vi "WildBugChilGru.vi"() -> ()   [LabVIEW 2014]
uses:
  <vilib>/Utility/miscctls.llb/LVPointTypeDef.ctl
  <vilib>/Utility/xml.llb/Write to XML File(string).vi
  <vilib>/Platform/browser.llb/Open URL in Default Browser (string).vi
  <vilib>/Instr/_visa.llb/VISA Configure Serial Port (Instr).vi
  <vilib>/Analysis/3filter.llb/IIR Filter (DBL).vi
  <vilib>/gmath/NI_Gmath.lvlib
  <vilib>/Analysis/NI_AALBase.lvlib
  <vilib>/ptbypt/NI_PtbyPt.lvlib
panel:
  out "Strecke [m]":dbl
  out "dT":dbl=3003.0
  out "Cyclecounter":dbl=3003.0
  out "Datum+Zeit":string="14.08.2020 22:16"
  out "n(Pmax)":dbl=5307.692307692308
  out "Pmax":dbl=17.77254327549455
  out "Lauf abgebrochen":bool
  out "Auto-Datei":string
  out "Auto-Gespeichert":bool
  in  "Auto-Pfad":path
  in  "Auto-Speichern":bool
  out "n(Rolle) [1/min]":dbl=3003.0
  in  "Fahrzeugdaten":string
  out "Ergebnis":string
  out "Pmax":string
  in  "Drucken":bool
  in  "Speichern":bool
  in  "Start":bool
  in  "Ende":bool
  in  "Spenden":bool
  in  "Registerkarte":T1(tab)
  in  "Zündung [Imp/U]":dbl=1.0 format="%#.2f"
  in  "Übersetzung ermitteln aus":T2(ring)
  in  "Getriebe [1:]":dbl=4.0 min=0.0001
  in  "Reifenumfang [m]":dbl=1.222 min=0.0001
  in  "Dauer [s]":u8=5
  in  "nKuWe/nRolle":dbl=20.0 format="%#.3f"
  in  "Lufttemperatur [°C]":dbl=23.3 format="%#.1g"
  in  "Luftdruck [mbar]":dbl=1013.45 min=0.0001
  in  "Messung Klimadaten":bool=TRUE
  in  "Filter Zündsignal":bool
  in  "v vom Gas [km/h]":u16=40
  in  "Gleitender Mittelwert":u8=35
  in  "Differenzenquotient":u8=12
  in  "n vom Gas [1/min]":u16=5000
  in  "Verlustmoment M1 [Nm] bei n1":dbl min=0.0
  in  "Rollendrehzahl n1 [1/min]":u16=1 min=1
  in  "Verlustmoment M0 [Nm] bei n = 0":dbl min=0.0
  in  "Rollengeber [Inkr/U]":u16=20 min=1
  in  "Rollenumfang [m]":dbl=0.5 min=0.0001
  in  "Rollenträgheit [kgm²]":dbl=2.0 min=0.0001
  in  "Rollendrehzahl aufzeichnen":bool
  in  "Überschrift Leistungsdiagramm":string
  in  "Recalc":bool
  in  "Leistung":bool=TRUE caption="Messung Klimadaten"
  out "Datenspeicher":T3={"Fahrzeugdaten"="§$", "Auto-Pfad"="14.08.2020 22:16|", "Rolle [Inkr/U]"=20, "Rollenumfang [m]"=0.5, "Rollenträgheit [kgm²]"=2.0, "Zündung [Imp/U]"=1.0, "Getriebe [1:]"=4.0, "Reifenumfang [m] "=1.222, "element"=0.0, "Gl. Mittelwert"=35, "Differenzenquotient"=12, 0, "dT [s]"=0.0163934426229508, "Strecke [m]"=326.5086065573754, "Lufttemperatur [°C]"=23.3, "Mv: n1 [1/min]"=1.0, "Luftdruck [mbar]"=1013.45, "nRolle"=array[1238 elements], "nWelle"=array[1238 elements], "ArrayReserve1"=array[1238 elements], "ArrayReserve2"=array[1238 elements], "Übersetzung ermitteln aus"=3, "[s]"=5.0, "Mv: M0 [Nm]"=0.0, "Mv: M1 [Nm]"=0.0, "n vom Gas [1/min]"=5000.0, "dT-Array [s]"=array[1238 elements], [], "Boolesch"=TRUE, "Serielle Schnittstelle"="COM6", "nKuWe/nRolle"=20.0, "v vom Gas [km/h]"=40.0}
  out "COM-Fehlerrate":string="0 / 0,0%"
  in  "Konfiguration:":bool
  out "Füllstand Lesepuffer":u64(slide)=1 scale=1.0..100.0
  out "Lesepuffer":string="\n"
  in  "Serielle Schnittstelle":refnum<visa-resource-name>="COM6"
  in  "Registerkarte 2":enum32{"Seite 1", "Seite 2"}(tab)
  out "Text Rolle":string="Rolle"
  out "Text Zündung":string="Zündung"
  in  "Reset Skalierung":bool
  out "Welle\n[1/min]":cluster{dbl, dbl}(knob) scale=0.0..14000.0
  out "Untersetzung\nermittelt":bool
  out "Hinterrad\n[km/h]":dbl(knob) scale=0.0..200.0
  out "XY-Graph":cluster{dbl[], dbl[]}[](graph)
  out "Untersetzung":dbl=1.0 format="%#.3f"
  out "Untersetzung-Graph":dbl(graph)=1.6366612111292962 caption="Untersetzung"
  # "Leistungsmessung:\n1. Drehzahl konstant halten\n2. START [F1]\n3. Drehzahl weiter halten\n4. bei GO: Vollgas\n5. vom Gas gehen"
  # "WildBugGruChil Dyno v2.0.9.1"
  # "Untersetzung aus:"
  # "Eingabe <> Messen"
  # "Tacho <> Leistung"
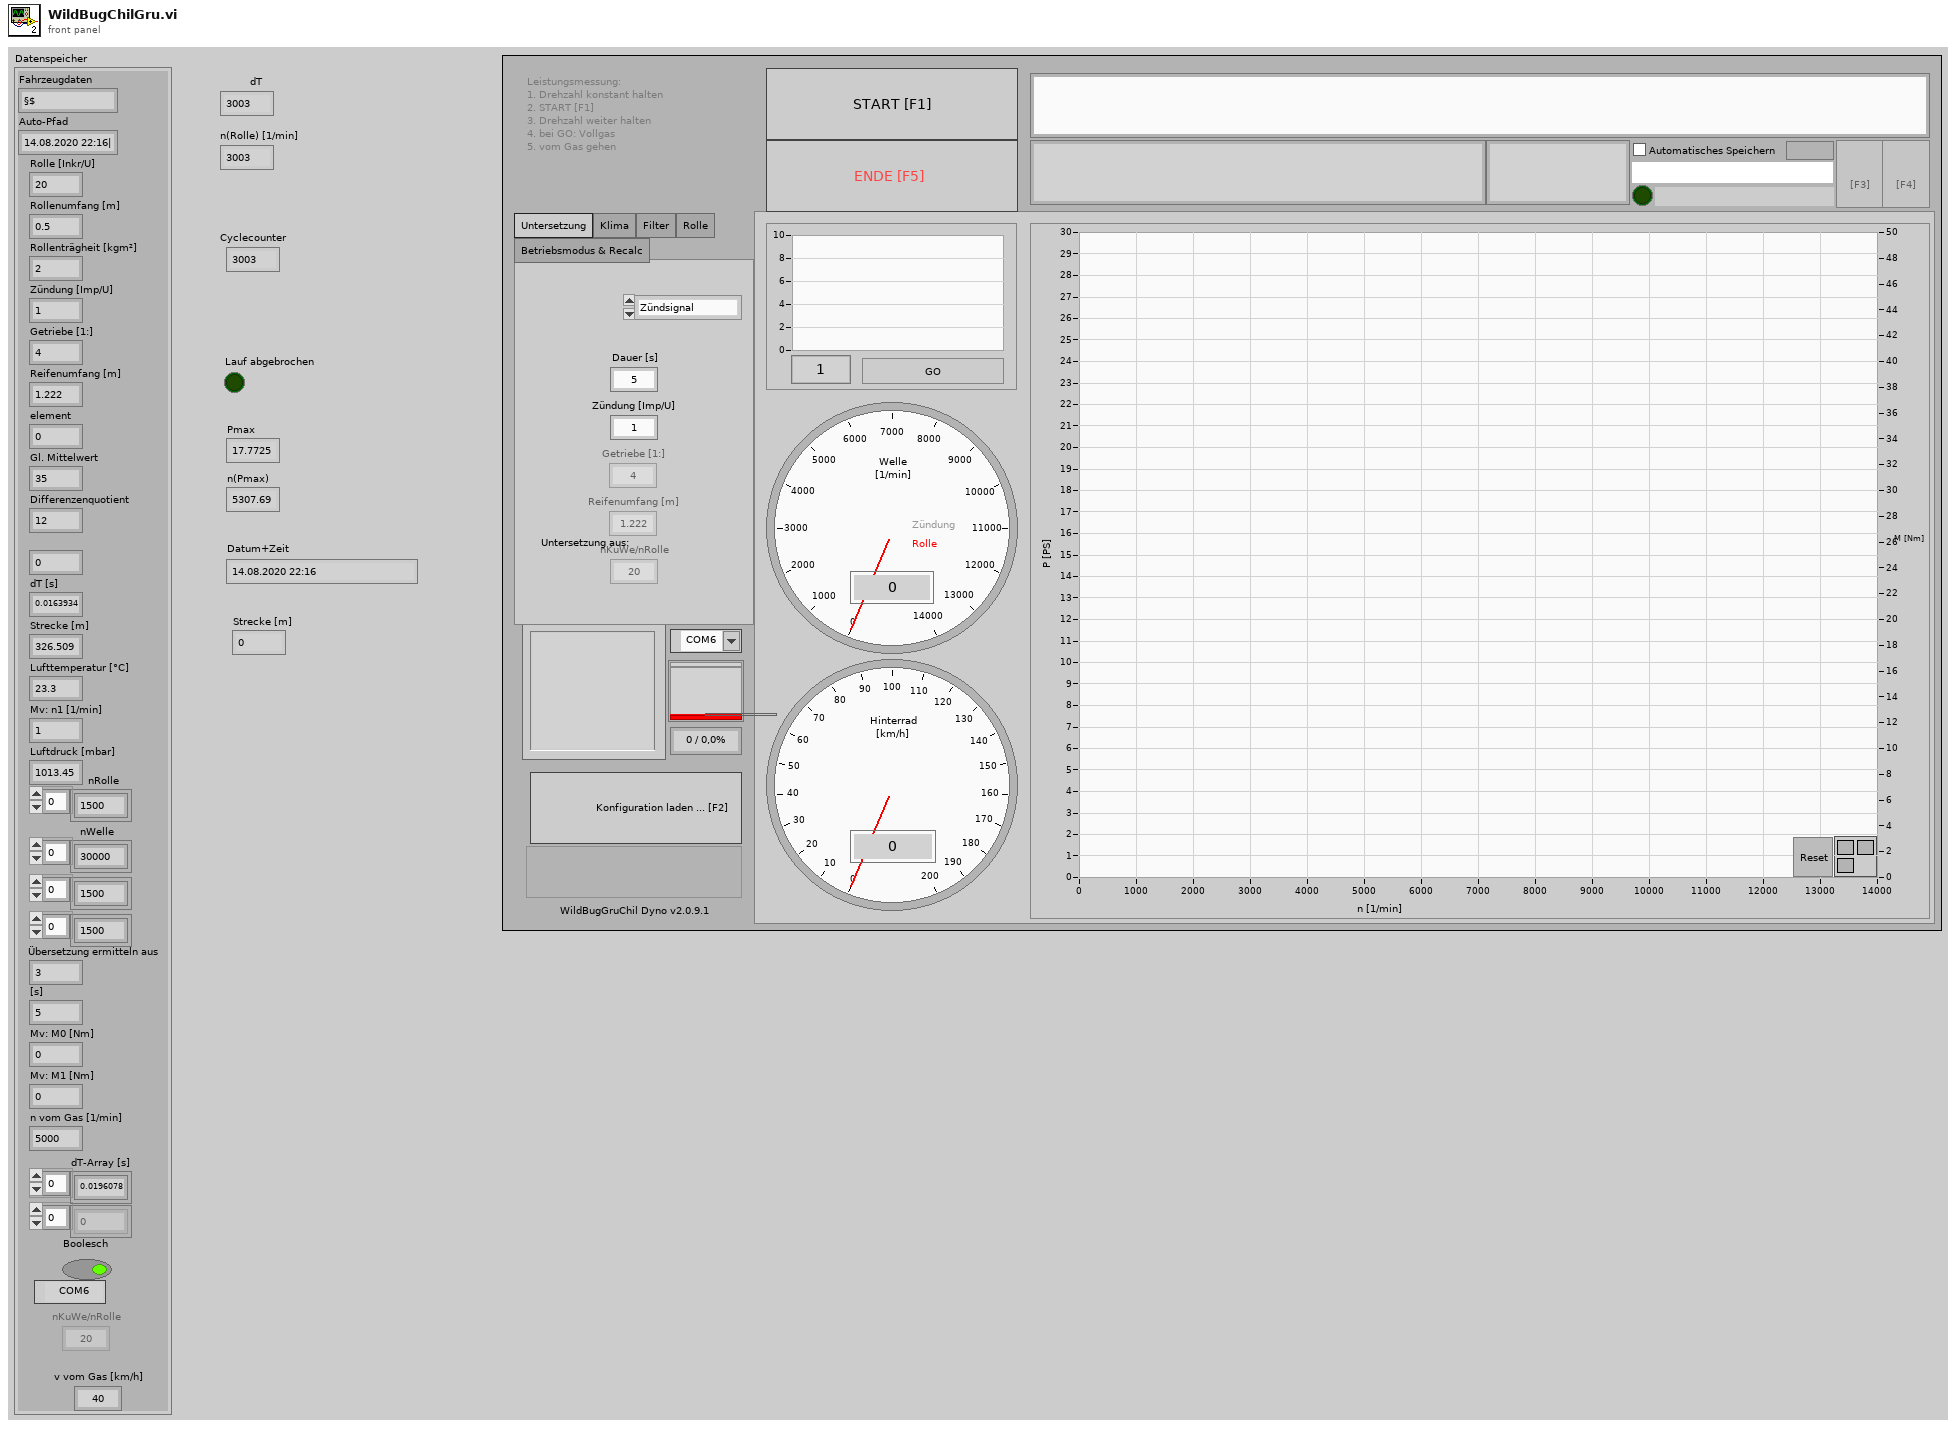
[diagram p1: front panel]
types:
  T1 = enum32{"Untersetzung", "Klima", "Filter", "Rolle", "Betriebsmodus & Recalc"}
  T2 = enum8{"Zündsignal", "Getriebe & Reifen", "nKuWe / nRolle", "Vario (km/h)"}
  T3 = cluster{"Fahrzeugdaten":string, "Auto-Pfad":string, "Rolle [Inkr/U]":u16, "Rollenumfang [m]":dbl, "Rollenträgheit [kgm²]":dbl, "Zündung [Imp/U]":dbl, "Getriebe [1:]":dbl, "Reifenumfang [m] ":dbl, "element":dbl, "Gl. Mittelwert":u8, "Differenzenquotient":u8, u8, "dT [s]":dbl, "Strecke [m]":dbl, "Lufttemperatur [°C]":dbl, "Mv: n1 [1/min]":dbl, "Luftdruck [mbar]":dbl, "nRolle":dbl[], "nWelle":dbl[], "ArrayReserve1":dbl[], "ArrayReserve2":dbl[], "Übersetzung ermitteln aus":u8, "[s]":dbl, "Mv: M0 [Nm]":dbl, "Mv: M1 [Nm]":dbl, "n vom Gas [1/min]":dbl, "dT-Array [s]":dbl[], i32[], "Boolesch":bool, "Serielle Schnittstelle":refnum<visa-resource-name>, "nKuWe/nRolle":dbl, "v vom Gas [km/h]":dbl}
  T4 = enum8{"Enabled", "Disabled", "Disabled and Grayed Out"}
  T5 = cluster{"Array (Ausgang)":dbl[], "Filtered X":dbl[]}
  T6 = cluster{"Array (Ausgang)":dbl[], "Filtered X":dbl[]}[]
  T7 = cluster{string, string, "Rollengeber [Inkr/U]":u16, "Rollenumfang [m]":dbl, "Rollenträgheit [kgm²]":dbl, "Zündung [Imp/U]":dbl, "Getriebe [1:]":dbl, "Reifenumfang [m] ":dbl, "mean value":dbl, "Gleitender Mittelwert":u8, "Differenzenquotient":u8, u8, dbl, "Strecke [m]":dbl, "Lufttemperatur [°C]":dbl, "Rollendrehzahl n1 [1/min]":u16, "Luftdruck [mbar]":dbl, dbl[], dbl[], dbl[], dbl[], "Übersetzung ermitteln aus":enum8{"Zündsignal", "Getriebe & Reifen", "nKuWe / nRolle", "Vario (km/h)"}, "Dauer [s]":u8, "Verlustmoment M0 [Nm] bei n = 0 ":dbl, "Verlustmoment M1 [Nm] bei n1":dbl, "n vom Gas [1/min]":u16, dbl[], i32[], "Messung Klimadaten":bool, "VISA-Referenz (Ausgang)":refnum<visa-resource-name>, "nKuWe/nRolle":dbl, "v vom Gas [km/h]":u16}
  T8 = typedef "LVPointTypeDef.ctl" = cluster{"Horizontal":i16, "Vertical":i16}
  T9 = enum32{"invalid app kind", "Development System", "Run Time System", "Student Edition", "Embedded LabVIEW", "Evaluation", "Custom"}
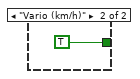
[diagram p3: hidden frame]
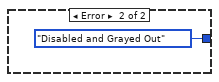
[diagram p5: hidden frame]
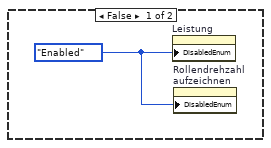
[diagram p6: hidden frame]
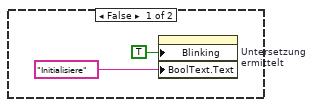
[diagram p7: hidden frame]
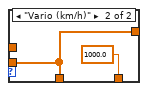
[diagram p13: hidden frame]
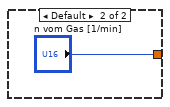
[diagram p14: hidden frame]
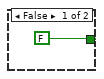
[diagram p15: hidden frame]
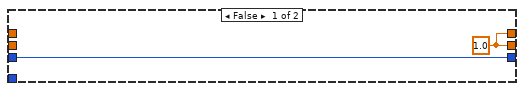
[diagram p18: hidden frame]
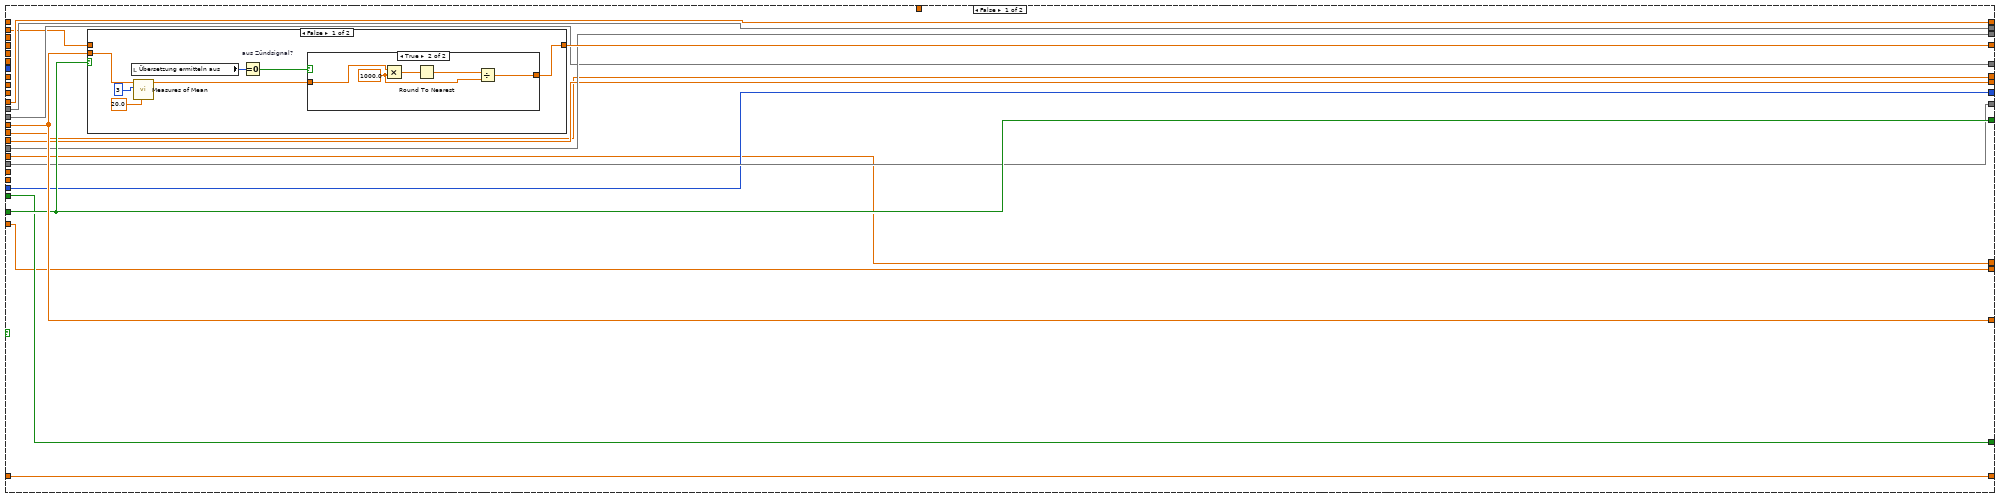
[diagram p19: hidden frame]
diagram:
  w2 = FALSE
  n1 = while {
    stop <- w12 stop-if-true
    n2 = local read "Rollendrehzahl aufzeichnen"() -> (w9:bool)
    n3 = Wait (ms)(milliseconds to wait=10) -> ()  [unwired: 1 out]
    n4 = Not(x=w9) -> (.not. x?=w8:bool)
    n5 = And(x="Leistung", y=w8) -> (x .and. y?=w6:bool)
    n6 = local read "Start"() -> (w13:bool)
    n7 = Not(x=w6) -> (.not. x?=w10:bool)
    n8 = case shown="True" w13 {
      tunnel: w6 -> [_ w48]
      frame False {
        w14 = T4."Enabled" ("Deaktiviert")
        n9 = property on="Leistung" class="Bool. (strikt)"("DisabledEnum"=w14) -> ()  [unwired: 2 in, 2 out]
        n10 = property on="Rollendrehzahl aufzeichnen" class="Bool. (strikt)"("DisabledEnum"=w14) -> ()  [unwired: 2 in, 2 out]
      }
      frame True {
        w28 = 0
        w29 = 0.0
        w31 = 0
        w35 = FALSE
        n11 = flat-sequence {
          tunnel: [w97] -> w80
          tunnel: [w96] -> w79
          tunnel: [w94] -> w78
          tunnel: w48 -> [w92]
          tunnel: [w91] -> w23
          tunnel: [w87] -> w20
          tunnel: w80 -> [w125]
          tunnel: w79 -> [w127]
          tunnel: [w119] -> w77
          tunnel: [w125] -> w76
          tunnel: [w127] -> w75
          tunnel: w78 -> [w126]
          tunnel: [w126] -> w74
          tunnel: [w117] -> w24
          tunnel: w23 -> [w117]
          tunnel: w20 -> [w116]
          tunnel: [w116] -> w19
          tunnel: [w143] -> w73
          tunnel: [w142] -> w47
          tunnel: [w141] -> w46
          tunnel: w77 -> [w143]
          tunnel: w76 -> [w139]
          tunnel: w75 -> [w138]
          tunnel: w74 -> [w140]
          tunnel: w24 -> [w134]
          tunnel: w19 -> [w135]
          tunnel: [w135] -> w18
          tunnel: [w134] -> w17
          tunnel: w73 -> [w152]
          tunnel: [w152] -> w72
          tunnel: [w151] -> w71
          tunnel: [w150] -> w70
          tunnel: [w148] -> w69
          tunnel: w47 -> [w151]
          tunnel: w46 -> [w150]
          tunnel: [w145] -> w22
          tunnel: w18 -> [w145]
          tunnel: w17 -> [w144]
          tunnel: [w144] -> w16
          tunnel: ["Gleitender Mittelwert"] -> w57
          tunnel: [w161] -> w58
          tunnel: [w160] -> w59
          tunnel: [w179] -> w60
          tunnel: [w173] -> w55
          tunnel: [w172] -> w56
          tunnel: [w180] -> w61
          tunnel: w72 -> [w180]
          tunnel: w71 -> [w175]
          tunnel: w70 -> [w174]
          tunnel: w69 -> [w179]
          tunnel: [w166] -> w45
          tunnel: [w167] -> w44
          tunnel: [w155] -> w41
          tunnel: [w154] -> w21
          tunnel: w22 -> [w154]
          tunnel: w16 -> [w153]
          tunnel: [w153] -> w15
          frame #0 {
            w102 = u16 0 items=["None", "XON/XOFF", "RTS/CTS", "XON/XOFF & RTS/CTS", "DTR/DSR", "XON/XOFF & DTR/DSR"] ("flow control (0:none)")
            w103 = u16 10 items=["1.0"=10, "1.5"=15, "2.0"=20] ("stop bits (10: 1 bit)")
            w95 = FALSE  # Enable Termination Char (T)
            w98 = u32 10000  # timeout (10sec)
            n12 = flat-sequence {
              tunnel: [w110] -> w90
              tunnel: [w109] -> w89
              tunnel: [w108] -> w88
              tunnel: [w113] -> w91
              tunnel: w90 -> [w115]
              tunnel: w89 -> [w114]
              tunnel: [w112] -> w87
              tunnel: w88 -> [w112]
              frame #0 {
                w109 = 0
                w110 = 4
                n13 = Open/Create/Replace File "Datei COM"(prompt="COM", operation (0:open)=w110, access (0:read/write)=w109) -> (refnum out=w108:refnum<file>)  [unwired: 3 in, 2 out]
              }
              frame #1 {
                n14 = Open/Create/Replace File "Datei LV-Interpretation"(prompt="LV-Interpretation", operation (0:open)=w115, access (0:read/write)=w114) -> (refnum out=w113:refnum<file>)  [unwired: 3 in, 2 out]
              }
            }
            n15 = And(x="Messung Klimadaten", y=w92) -> (x .and. y?=w94:bool)
            n16 = call-poly "VISA Configure Serial Port"("VISA resource name"="Serielle Schnittstelle", "timeout (10sec)"=w98, "Enable Termination\nChar (T)"=w95, "baud rate (9600)"=u32 115200 ("baudrate (250000)"), "data bits (8)"=u16 8, "parity (0:none)"=enum16{"None", "Odd", "Even", "Mark", "Space"}."None", "stop bits (10: 1 bit)"=w103, "flow control (0:none)"=w102) -> ("VISA resource name out"=w100:refnum<visa-resource-name>, "error out"=w99:errorcluster)  [unwired: 6 in]
            n17 = VISA Clear(VISA resource name=w100, error in (no error)=w99) -> (VISA resource name out=w97:refnum<visa-resource-name>, error out=w96:errorcluster)
          }
          frame #1 {
            w118 = FALSE
            w120 = T4."Disabled and Grayed Out" ("Deaktiviert")
            w128 = 0.0  # Graphen löschen
            w119 = ""
            n18 = case shown="True" w126 {
              frame False {
                n19 = property on="Untersetzung\nermittelt" class="Bool. (strikt)"("Blinking"=TRUE ("Blinkend"), "BoolText.Text"="Initialisiere" ("Beschriftung.Text")) -> ()  [unwired: 2 in, 2 out]
              }
              frame True {
                n20 = Wait (ms)(milliseconds to wait=u32 2000 ("Zu wartende ms")) -> ()  [unwired: 1 out]
                n21 = property on="Untersetzung\nermittelt" class="Bool. (strikt)"("Blinking"=TRUE ("Blinkend"), "BoolText.Text"="Lese Klimadaten" ("Beschriftung.Text")) -> ()  [unwired: 2 in, 2 out]
              }
            }
            n22 = Build Array(w128) -> (w121:dbl[])
            n23 = property on="Auto-Gespeichert" class="Bool. (strikt)"("Value"=w118) -> ()  [unwired: 2 in, 2 out]
            n24 = property on="Lauf abgebrochen" class="Bool. (strikt)"("Value"=w118) -> ()  [unwired: 2 in, 2 out]
            n25 = property on="Untersetzung-Graph" class="SVDiagr (strikt)"("History Data"=w121) -> ()  [unwired: 2 in, 2 out]
            n26 = property on="Drucken" class="Bool. (strikt)"("DisabledEnum"=w120) -> ()  [unwired: 2 in, 2 out]
            n27 = property on="Übersetzung ermitteln aus" class="Enum (strikt)"("DisabledEnum"=w120) -> ()  [unwired: 2 in, 2 out]
            n28 = property on="Konfiguration:" class="Bool. (strikt)"("DisabledEnum"=w120) -> ()  [unwired: 2 in, 2 out]
            n29 = property on="Ende" class="Bool. (strikt)"("DisabledEnum"=w120) -> ()  [unwired: 2 in, 2 out]
            n30 = property on="Leistung" class="Bool. (strikt)"("DisabledEnum"=w120) -> ()  [unwired: 2 in, 2 out]
            n31 = property on="Speichern" class="Bool. (strikt)"("DisabledEnum"=w120) -> ()  [unwired: 2 in, 2 out]
            n32 = property on="Rollendrehzahl aufzeichnen" class="Bool. (strikt)"("DisabledEnum"=w120) -> ()  [unwired: 2 in, 2 out]
            n33 = local write "Pmax"(w119) -> ()
            n34 = local write "COM-Fehlerrate"(w119) -> ()
            n35 = local write "Ergebnis"(w119) -> ()
            n36 = Bundle(w121, w121) -> (w123:cluster{dbl[], dbl[]})  [unwired: 1 in]
            n37 = Bundle(w121, w121) -> (w122:cluster{dbl[], dbl[]})  [unwired: 1 in]
            n38 = Build Array(w123, w122) -> (w124:cluster{dbl[], dbl[]}[])
            n39 = local write "Auto-Datei"(w119) -> ()
            n40 = local write "XY-Graph"(w124) -> ()
          }
          frame #2 {
            n41 = control-ref of="Lufttemperatur [°C]"() -> (w136:refnum<vi>)
            n42 = control-ref of="Luftdruck [mbar]"() -> (w137:refnum<vi>)
            n43 = call "MessungKlimadaten(SubVI).vi"("Datei LV-Interpretation"=w134, "Datei COM"=w135, "Boolesch"=w140, "Fehler (Eingang, kein Fehler)"=w138, "VISA resource name out"=w139, "Lufttemperatur [°C] (Eingang)"=w136, "Luftdruck [mbar] (Eingang)"=w137) -> ("Fehler (Ausgang)"=w141:errorcluster, "VISA-Referenz (Ausgang)"=w142:refnum<visa-resource-name>)  [unwired: 3 in]
          }
          frame #3 {
            n44 = Wait (ms)(milliseconds to wait=u32 2000 ("Zu wartende ms")) -> ()  [unwired: 1 out]
            n45 = call "KorrekturfaktorDin70020 (SubVI).vi"("Lufttemperatur [°C]"="Lufttemperatur [°C]", "Luftdruck [mbar]"="Luftdruck [mbar]") -> ("Korrekturfaktor"=w148:dbl)  [unwired: 9 in]
          }
          frame #4 {
            w156 = 0
            n46 = property on="XY-Graph" class="XYGraph (strikt)"("ActYScl"=w156, "YScale.ScaleFit"=w156, "ActYScl"=1, "YScale.ScaleFit"=w156, "XScale.ScaleFit"=w156, "Smooth Update"=TRUE ("Kontinuierliche Aktualisierung")) -> ()  [unwired: 2 in, 2 out]
            n47 = Concatenate Strings("m" ("String"), "\n") -> (w178:string)
            n48 = VISA Write(VISA resource name=w175, write buffer=w178, error in (no error)=w174) -> (VISA resource name out=w172:refnum<visa-resource-name>, error out=w173:errorcluster)  [unwired: 1 out]
            n49 = local read "Differenzenquotient"() -> (w170:u8)
            n50 = property on="Untersetzung\nermittelt" class="Bool. (strikt)"("Blinking"=FALSE ("Blinkend")) -> ()  [unwired: 2 in, 2 out]
            n51 = Divide(x="Gleitender Mittelwert", y=2) -> (x/y=w165:dbl)
            n52 = Round Toward -Infinity(1:w165) -> (0:w155:dbl)
            n53 = call <vilib>:"Smoothing Filter Coefficients.vi"("shape"=0, "half-width"=w170, "type"=0) -> ("forward coefficients"=w167:dbl[], "reverse coefficients"=w166:dbl[])  [unwired: 6 in, 1 out]
            n54 = call <vilib>:"Smoothing Filter Coefficients.vi"("shape"=1, "half-width"=w155, "type"=0) -> ("forward coefficients"=w161:dbl[], "reverse coefficients"=w160:dbl[])  [unwired: 6 in, 1 out]
          }
        }
        n55 = Initialize Array(0.0 ("y"), 0) -> (w32:dbl[])
        n56 = Initialize Array(w28, w28) -> (w27:i32[])
        n57 = while {
          tunnel: w56 -> [w382]
          tunnel: w55 -> [w381]
          shift-right: [w426] -> _
          shift-left: w61 -> [w388]
          shift-right: [w339] -> _
          shift-left: w29 -> [w425]
          shift-right: [w421] -> _
          shift-left: w29 -> [w424]
          shift-right: [w391] -> _
          shift-left: w29 -> [w423]
          shift-right: [w355] -> _
          shift-left: w31 -> [w422]
          shift-right: [w395] -> w65
          shift-left: w29 -> [w376]
          shift-right: [w372] -> w63
          shift-left: w29 -> [w336]
          shift-right: [w392] -> _
          shift-left: w32 -> [w418]
          shift-right: [w375] -> _
          shift-left: w35 -> [w371]
          shift-right: [w415] -> w64
          shift-left: w32 -> [w413]
          shift-right: [w414] -> _
          shift-left: w32 -> [w328]
          shift-right: [w367] -> w37
          shift-left: w32 -> [w412]
          shift-right: [w409] -> _
          shift-left: w32 -> [w410]
          shift-right: [w408] -> w49
          shift-left: w32 -> [w411]
          shift-right: [w366] -> w38
          shift-left: w32 -> [w330]
          shift-right: [w365] -> w39
          shift-left: w32 -> [w331]
          tunnel: [w407] -> w68
          shift-right: [w403] -> w67
          shift-left: w31 -> [w405]
          tunnel: [w406] -> w52
          tunnel: [w370] -> w66
          tunnel: ["Rollenumfang [m]"] -> w26
          shift-right: [w402] -> _
          shift-left: w35 -> [w380]
          shift-right: [w396] -> _
          shift-left: -5 -> [w401]
          shift-right: [w397] -> _
          shift-left: w29 -> [w400]
          shift-right: [w398] -> _
          shift-left: w29 -> [w399]
          shift-right: [w379] -> w25
          shift-left: w32 -> [w394]
          shift-right: [w325] -> _
          shift-left: _ -> [w390]
          shift-right: [w393] -> w62
          shift-left: w27 -> [w389]
          tunnel: [w387] -> w53
          tunnel: w60 -> [w341]
          tunnel: w59 -> [w383]
          tunnel: w58 -> [w364]
          tunnel: w57 -> [w340]
          tunnel: w45 -> [w378]
          tunnel: w44 -> [w377]
          shift-right: [w357] -> w42
          shift-left: w32 -> [w359]
          shift-right: [w356] -> w36
          shift-left: w32 -> [w329]
          tunnel: w41 -> [w348]
          tunnel: [w341] -> w40
          tunnel: w21 -> [w323]
          tunnel: w15 -> [w322]
          i -> [w361]
          stop <- w407 stop-if-true
          w354 = 3  # Vario(km/h)
          n58 = property class="Instr"(reference=w382, error in=w381) -> (reference out=w386:refnum<visa-resource-name>, error out=w385:errorcluster, "Serial Settings:Number of Bytes at Serial Port"=w344:u32)
          n59 = Greater?(x=w344, y=u32 1 ("min. Bytes")) -> (0:w345:bool)
          n60 = control-ref of="Füllstand Lesepuffer"() -> (w369:refnum<vi>)
          n61 = Select(t=w344, s=w345, f=u32 0 ("Bytes at Port")) -> (s? t:f=w343:u32)
          n62 = call "Stringhandling(SubVI)0.0.2.vi"("Slide (Eingang)"=w369, "Numerisch (Eingang)"=w422, "VISA-Referenz (Eingang)"=w386, "MessFrequenz [Hz]"=w423, "Bytes at Port"=w343, "Fehler (Eingang, kein Fehler)"=w385, "Cyclecounter (Eingang)"=w390, "Rolle[Hz]"=w424, "Datei COM"=w323, "String (Eingang)"=w388, "Zündung [Hz] (Eingang)"=w425, "Datei LV-Interpretation"=w322) -> ("Lesepuffer"=→"Lesepuffer":string, "Numerisch (Ausgang)"=w355:i32, "String (Ausgang)"=w426:string, "VISA-Referenz (Ausgang)"=w387:refnum<visa-resource-name>, "Zündung [Hz] (Ausgang)"=w338:dbl, "Rolle [Hz]"=w421:dbl, "Messfrequenz [Hz]"=w391:dbl, "Cyclecounter (Ausgang)"=w325:i32, "Fehler (Ausgang)"=w406:errorcluster)  [unwired: 7 in]
          "Füllstand Lesepuffer" <- w355
          "Cyclecounter" <- w325
          n63 = local read "Übersetzung ermitteln aus"() -> (w353:T2)
          n64 = Not Equal?(x=w354, y=w353) -> (x != y?=w351:bool)
          n65 = And(x="Filter Zündsignal", y=w351) -> (x .and. y?=w349:bool)
          n66 = Select(t=w348, s=w349, f=0) -> (s? t:f=w337:dbl)
          n67 = call <vilib>:"Median Filter PtByPt.vi"("initialize"=TRUE, "rank"=w337, "x"=w338) -> ("Filtered x"=w339:dbl)  [unwired: 1 in, 1 out]
          n68 = Not Equal?(x=w390, y=w325) -> (x != y?=w326:bool)
          n69 = case "Case-Struktur" shown="True" w326 {
            tunnel: w339 -> [w699 w720]
            tunnel: w421 -> [w698 w719]
            tunnel: [w699 w708] -> w420
            tunnel: [w698 w705] -> w419
            tunnel: w391 -> [_ w715]
            tunnel: w376 -> [w697 _]
            tunnel: [w697 w703] -> w395
            tunnel: w336 -> [_ w706]
            tunnel: "Rollenumfang [m]" -> [_ w718]
            tunnel: w353 -> [_ w712]
            frame False {
            }
            frame True {
              w723 = 60.0 ("y")
              n70 = Reciprocal "Abtastzeit [s]"(x=w715) -> (1/x=w703:dbl)
              "dT" <- w703
              n71 = Divide "R [1/s]"(x=w719, y="Rollengeber [Inkr/U]") -> (x/y=w707:dbl)
              n72 = Divide(x=w720, y="Zündung [Imp/U]") -> (x/y=w722:dbl)
              n73 = Multiply "[m/s]"(x=w707, y=w718) -> (x*y=w704:dbl)
              n74 = Multiply(x=w704, y=w703) -> (x*y=w700:dbl)
              n75 = Multiply "nZ gemessen [1/min]"(x=w722, y=w723) -> (x*y=w708:dbl)
              n76 = Multiply "nR [1/min]"(x=w723, y=w707) -> (x*y=w705:dbl)
              "n(Rolle) [1/min]" <- w705
              n77 = local read "Strecke [m]"() -> (w701:dbl)
              n78 = Multiply "nZ berechnet [1/min]"(x=w706, y=w705) -> (x*y=w710:dbl)
              n79 = case shown="Standard" w712 {
                tunnel: [w725 w726] -> w711
                tunnel: w710 -> [w725 w727]
                tunnel: [w724 w727] -> w709
                tunnel: w708 -> [w724 w726]
                frame Default {
                }
                frame "Vario (km/h)" {
                }
              }
              n80 = Add(x=w701, y=w700) -> (x+y=→"Strecke [m]":dbl)
              n81 = Bundle(w711, w709) -> (→"Welle\n[1/min]":cluster{dbl, dbl})  [unwired: 1 in]
              n82 = Multiply ("[km/h]")(x=w704, y=3.6) -> (x*y=→"Hinterrad\n[km/h]":dbl)
            }
          }
          n83 = case shown="True" w326 {
            tunnel: w401 -> [w464 w475]
            tunnel: [w464 w487] -> w396
            tunnel: w400 -> [w463 w486]
            tunnel: [w463 w472] -> w397
            tunnel: w399 -> [w462 w485]
            tunnel: [w462 w473] -> w398
            tunnel: w325 -> [_ w471]
            tunnel: w389 -> [w461 w470]
            tunnel: [w461 w474] -> w393
            frame False {
            }
            frame True {
              n84 = Build Array (concatenate)(w470, w471) -> (w474:i32[])
              n85 = Greater Or Equal To 0?(x=w475) -> (x >= 0?=w476:bool)
              n86 = case shown="True" w476 {
                tunnel: [w488 w499] -> w472
                tunnel: [w488 w500] -> w473
                tunnel: [w489 w491] -> w487
                tunnel: w486 -> [_ w493]
                tunnel: w485 -> [_ w501]
                tunnel: w471 -> [w489 w490]
                tunnel: w475 -> [_ w491]
                frame False {
                  w488 = 1.0
                }
                frame True {
                  w497 = 65536.0
                  n87 = Add(x=w491, y=w493) -> (x+y=w492:dbl)
                  n88 = Divide(x=w492, y=w497) -> (x/y=w502:dbl)
                  n89 = Increment(x=w501) -> (x+1=w500:dbl)
                  n90 = Round Toward -Infinity(1:w502) -> (0:w498:dbl)
                  n91 = Multiply(x=w498, y=w497) -> (x*y=w496:dbl)
                  n92 = Add(x=w496, y=w490) -> (x+y=w495:dbl)
                  n93 = Increment(x=w495) -> (x+1=w494:dbl)
                  n94 = Subtract(x=w494, y=w491) -> (x-y=w499:dbl)
                }
              }
              n95 = Subtract(x=w472, y=w473) -> (x-y=w467:dbl)
              n96 = Decrement(x=w467) -> (x-1=w466:dbl)
              n97 = Max & Min(x=0, y=w466) -> (max(x,y)=w465:dbl)  [unwired: 1 out]
              n98 = Divide(x=w465, y=w472) -> (x/y=w479:dbl)
              n99 = Greater Than 0?(x=w465) -> (x > 0?=w469:bool)
              n100 = Select(t=u32 16711680, s=w469, f=u32 0) -> (s? t:f=w480:u32)
              n101 = Multiply(x=w479, y=100.0) -> (x*y=w477:dbl)
              n102 = property on="COM-Fehlerrate" class="Str"("Text.TextColor"=w480) -> ()  [unwired: 2 in, 2 out]
              n103 = Format Into String(format string="%d / %.1f%%" ("Format-String"), w465, w477) -> (resulting string=→"COM-Fehlerrate":string)  [unwired: 2 in, 1 out]
            }
          }
          n104 = case shown="\"Vario (km/h)\"" w353 {
            tunnel: [w453 "n vom Gas [1/min]"] -> w370
            frame "Vario (km/h)" {
              n105 = local read "Rollenumfang [m]"() -> (w454:dbl)
              n106 = Divide(x="v vom Gas [km/h]", y=w454) -> (x/y=w452:dbl)
              n107 = Multiply(x=w452, y=16.66666667) -> (x*y=w453:dbl)
            }
            frame Default {
            }
          }
          n108 = case shown="True" w326 {
            tunnel: w420 -> [_ w555]
            tunnel: w419 -> [_ w608]
            tunnel: "Rollenumfang [m]" -> [_ w609]
            tunnel: [w516 w538] -> w372
            tunnel: w336 -> [w505 w538]
            tunnel: w371 -> [w517 w557]
            tunnel: w418 -> [w518 w612]
            tunnel: [w517 w584] -> w375
            tunnel: [w518 w611] -> w392
            tunnel: w383 -> [_ w554]
            tunnel: w364 -> [_ w553]
            tunnel: [w515 w535] -> w415
            tunnel: [w514 w536] -> w414
            tunnel: w413 -> [w515 w607]
            tunnel: w328 -> [w514 _]
            tunnel: w340 -> [_ w552]
            tunnel: [w513 w542] -> w367
            tunnel: w412 -> [w513 _]
            tunnel: [w512 w565] -> w409
            tunnel: w410 -> [w512 _]
            tunnel: [w511 w549] -> w408
            tunnel: w411 -> [w511 _]
            tunnel: [w510 w543] -> w366
            tunnel: w330 -> [w510 _]
            tunnel: [w509 w601] -> w365
            tunnel: w331 -> [w509 _]
            tunnel: w341 -> [_ w551]
            tunnel: w405 -> [w508 w595]
            tunnel: w370 -> [_ w586]
            tunnel: [w508 w594] -> w403
            tunnel: w380 -> [w507 w591]
            tunnel: [w507 w590] -> w402
            tunnel: w395 -> [_ w589]
            tunnel: [w506 w559] -> w379
            tunnel: w394 -> [w506 w588]
            tunnel: w378 -> [_ w572]
            tunnel: w377 -> [_ w571]
            tunnel: w359 -> [w504 w556]
            tunnel: [w504 w537] -> w357
            tunnel: [w503 w533] -> w356
            tunnel: w329 -> [w503 _]
            tunnel: w348 -> [_ w534]
            frame False {
              n109 = case shown="False" w517 {
                tunnel: w518 -> [w525 _]
                tunnel: [w519 w532] -> w516
                tunnel: w505 -> [_ w532]
                frame False {
                  n110 = local read "Übersetzung ermitteln aus"() -> (w522:T2)
                  n111 = call <vilib>:"Measures of Mean.vi"("percent (trim)"=20.0, "type"=3, "x array"=w525) -> ("mean value"=w520:dbl)  [unwired: 7 in, 1 out]
                  n112 = Equal To 0? "aus Zündsignal?"(x=w522) -> (x = 0?=w521:bool)
                  n113 = case shown="True" w521 {
                    tunnel: w520 -> [w526 w531]
                    tunnel: [w526 w527] -> w519
                    frame False {
                    }
                    frame True {
                      w528 = 1000.0
                      n114 = Multiply(x=w531, y=w528) -> (x*y=w530:dbl)
                      n115 = Round To Nearest(number=w530) -> (nearest integer value=w529:dbl)
                      n116 = Divide(x=w529, y=w528) -> (x/y=w527:dbl)
                    }
                  }
                }
                frame True {
                }
              }
            }
            frame True {
              w598 = 0.00135962  # [W] in [PS]
              w603 = 0.10471975511965978  # 2*Pi/60
              # "Einzelne Ausreisser (Zündsignal) werden\nam besten mit Median-Filter eliminiert"
              n117 = Not(x=w557) -> (.not. x?=w562:bool)
              n118 = local read "Leistung"() -> (w561:bool)
              n119 = Or(x=w561, y=w562) -> (x .or. y?=w560:bool)
              n120 = Square(x=w538) -> (x^2=w602:dbl)
              n121 = local read "Übersetzung ermitteln aus"() -> (w563:T2)
              n122 = case shown="False" w560 {
                tunnel: w608 -> [_ w624]
                tunnel: w607 -> [w614 w623]
                tunnel: w589 -> [_ w622]
                tunnel: w588 -> [w615 w621]
                tunnel: [w614 w620] -> w535
                tunnel: [w615 w619] -> w559
                tunnel: w556 -> [w613 w618]
                tunnel: [w613 w617] -> w537
                tunnel: w555 -> [_ w616]
                frame False {
                }
                frame True {
                  n123 = Build Array (concatenate) "nRolle in Array einf."(w623, w624) -> (w620:dbl[])
                  n124 = Build Array (concatenate) "dT in Array einf."(w621, w622) -> (w619:dbl[])
                  n125 = Build Array (concatenate) "nWelle in Array einf."(w618, w616) -> (w617:dbl[])
                }
              }
              n126 = Divide(x="Rollenträgheit [kgm²]", y=w602) -> (x/y=w550:dbl)
              n127 = case shown="\"Zündsignal\"" w563 {
                tunnel: w555 -> [w689 _ _ _]
                tunnel: w608 -> [w688 _ _ _]
                tunnel: [w687 w693 "nKuWe/nRolle" 1.0] -> w610
                tunnel: w609 -> [_ w694 _ _]
                frame "Zündsignal" {
                  n128 = Divide(x=w689, y=w688) -> (x/y=w687:dbl)
                }
                frame "Getriebe & Reifen" {
                  n129 = Divide(x=w694, y="Reifenumfang [m]") -> (x/y=w692:dbl)
                  n130 = Multiply(x=w692, y="Getriebe [1:]") -> (x*y=w693:dbl)
                }
                frame "nKuWe / nRolle" {
                }
                frame "Vario (km/h)" {
                }
              }
              n131 = Multiply(x=w551, y=w550) -> (x*y=w548:dbl)
              n132 = local read "Differenzenquotient"() -> (w570:u8)
              n133 = Multiply(x=2, y=w570) -> (x*y=w568:i32)
              n134 = Increment(x=w568) -> (x+1=w566:i32)
              n135 = Index Array(array=w535, index=1 ("Index")) -> (element=w582:dbl)
              n136 = Index Array(array=w559, index=1 ("Index")) -> (element=w576:dbl)
              n137 = Initialize Array(w582, w552) -> (w581:dbl[])
              n138 = Initialize Array(w576, w566) -> (w574:dbl[])
              n139 = Insert Into Array(array=w535, index=0 ("Index"), new element=w581) -> (w579:dbl[])
              n140 = Insert Into Array(array=w559, index=0 ("Index"), new element=w574) -> (w573:dbl[])
              n141 = call-poly <vilib>:"IIR Filter.vi"("Forward Coefficients"=w553, "Reverse Coefficients"=w554, "X"=w579) -> ("Filtered X"=w578:dbl[])  [unwired: 1 in, 1 out]
              n142 = call-poly <vilib>:"IIR Filter.vi"("Forward Coefficients"=w571, "Reverse Coefficients"=w572, "X"=w573) -> ("Filtered X"=w567:dbl[])  [unwired: 1 in, 1 out]
              n143 = case shown="False" w557 {
                selector: w557 -> [_ w686]
                tunnel: w610 -> [w674 _]
                tunnel: w612 -> [w676 w685]
                tunnel: [w671 w686] -> w606
                tunnel: [w675 w685] -> w611
                tunnel: w591 -> [w673 w684]
                tunnel: [w671 w684] -> w590
                tunnel: w563 -> [w670 _]
                frame False {
                  n144 = Build Array (concatenate)(w676, w674) -> (w675:dbl[])
                  n145 = case shown="\"Zündsignal\"" w670 {
                    tunnel: ["Dauer [s]" 0.0 ("Dauer [s]")] -> w672
                    frame "Zündsignal" {
                      n146 = property on="Untersetzung\nermittelt" class="Bool. (strikt)"("Blinking"=TRUE ("Blinkend"), "BoolText.Text"="Ermittle Übersetzung" ("Boolescher Text.Text")) -> ()  [unwired: 2 in, 2 out]
                    }
                    frame Default {
                    }
                  }
                  n147 = call "Verstrichene Zeit"("Time Target (s)"=w672, "Reset"=w673) -> ("Time has Elapsed"=w671:bool)  [unwired: 10 in, 7 out]
                  n148 = case shown="True" w671 {
                    frame False {
                    }
                    frame True {
                      n149 = property on="Untersetzung\nermittelt" class="Bool. (strikt)"("Blinking"=FALSE ("Blinkend"), "BoolText.Text"="Go" ("Boolescher Text.Text")) -> ()  [unwired: 2 in, 2 out]
                      n150 = property on="Strecke [m]" class="DigWert (strikt)"("Value"=0.0) -> ()  [unwired: 2 in, 2 out]
                    }
                  }
                  "Untersetzung-Graph" <- w674
                }
                frame True {
                }
              }
              n151 = Array Subset "Rolle gefiltert [1/min]"(array=w578, index=w552) -> (w536:dbl[])  [unwired: 1 in]
              n152 = Array Subset "dT gefiltert [s]"(array=w567, index=w566) -> (w564:dbl[])  [unwired: 1 in]
              n153 = Array Size "Array-Größe"(array=w536) -> (size(s)=w604:i32)
              n154 = Greater?(x=w604, y=w552) -> (0:w605:bool)
              n155 = call <vilib>:"Median Filter.vi"("right rank"=w534, "left rank"=w534, "X"=w537) -> ("Filtered X"=w533:dbl[])  [unwired: 7 in, 1 out]
              n156 = Multiply "* i"(x=w536, y=w538) -> (x*y=w542:dbl[])
              n157 = Multiply(x=w542, y=w603) -> (x*y=w565:dbl[])
              n158 = And(x=w606, y=w605) -> (x .and. y?=w584:bool)
              n159 = Array Size "Array-Größe"(array=w565) -> (size(s)=w558:i32)
              n160 = Decrement(x=w558) -> (x-1=w596:i32)
              n161 = Select(t=w586, s=w584, f=1000000.0) -> (s? t:f=w587:dbl)
              n162 = Initialize Array(0.0 ("y"), 0) -> (w544:dbl[])
              n163 = for {
                N: w558 -> [_]
                tunnel: "Differenzenquotient" -> [w647]
                tunnel: w565 -> [w654]
                tunnel: w596 -> [w646]
                shift-right: [w651] -> w549
                shift-left: w544 -> [w652]
                tunnel: w542 -> [w629] mode=indexing
                tunnel: w595 -> [w639]
                tunnel: w587 -> [w649]
                tunnel: [w640] -> w594
                tunnel: w557 -> [w638]
                tunnel: w564 -> [w635] mode=indexing
                tunnel: "Rollendrehzahl n1 [1/min]" -> [w632]
                tunnel: "Verlustmoment M1 [Nm] bei n1" -> [w631]
                tunnel: "Verlustmoment M0 [Nm] bei n = 0" -> [w630]
                shift-right: [w628] -> w541
                shift-left: w544 -> [w627]
                tunnel: w536 -> [w625] mode=indexing
                i -> [w636]
                stop <- w633 stop-if-true
                # "Beschleunigung a(i) berechnen solange bis n(i) > nSchwelle & a(i) < 0"
                n164 = call "Verlustmoment (SubVI).vi"("n [1/min"=w625, "Verlustmoment M0 [Nm] bei n = 0"=w630, "Verlustmoment M1 [Nm] bei n1"=w631, "Rollendrehzahl n1 [1/min]"=w632) -> ("Mv"=w626:dbl)  [unwired: 7 in]
                n165 = Subtract(x=w646, y=w647) -> (x-y=w648:i32)
                n166 = Multiply(x=w635, y=2.0) -> (x*y=w637:dbl)
                n167 = Subtract(x=w636, y=w647) -> (x-y=w667:i32)
                n168 = Add(x=w636, y=w647) -> (x+y=w661:i32)
                n169 = Greater Or Equal?(x=w636, y=w647) -> (x >= y?=w643:bool)
                n170 = Less Or Equal?(x=w636, y=w648) -> (x <= y?=w644:bool)
                n171 = Greater?(x=w629, y=w649) -> (0:w650:bool)
                n172 = Max & Min(x=w646, y=w661) -> (min(x,y)=w662:i32)  [unwired: 1 out]
                n173 = Max & Min(x=w667, y=0) -> (max(x,y)=w665:i32)  [unwired: 1 out]
                n174 = Subtract(x=w662, y=w636) -> (x-y=w663:i32)
                n175 = Subtract(x=w636, y=w665) -> (x-y=w664:i32)
                n176 = Max & Min(x=w664, y=w663) -> (min(x,y)=w655:i32)  [unwired: 1 out]
                n177 = Add(x=w636, y=w655) -> (x+y=w660:i32)
                n178 = Subtract(x=w636, y=w655) -> (x-y=w659:i32)
                n179 = Multiply(x=w655, y=w637) -> (x*y=w653:dbl)
                n180 = Index Array(array=w654, index=w660) -> (element=w657:dbl)
                n181 = Index Array(array=w654, index=w659) -> (element=w658:dbl)
                n182 = Subtract(x=w657, y=w658) -> (x-y=w656:dbl)
                n183 = Divide(x=w656, y=w653) -> (x/y=w645:dbl)
                n184 = Less Than 0?(x=w645) -> (x < 0?=w642:bool)
                n185 = Less Or Equal To 0?(x=w639) -> (x <= 0?=w641:bool)
                n186 = Build Array (concatenate)(w652, w645) -> (w651:dbl[])
                n187 = Compound Arithmetic op=AND "n(i) > nSchwelle\n& a(i) < 0"(w642, w650, w641, w643, w644, w638) -> (w633:bool)
                n188 = case shown="False" w633 {
                  tunnel: w636 -> [_ w669]
                  tunnel: [w668 w669] -> w640
                  tunnel: w639 -> [w668 _]
                  frame False {
                  }
                  frame True {
                  }
                }
                n189 = Build Array (concatenate) "Mv Rolle"(w627, w626) -> (w628:dbl[])
              }
              n190 = Divide ": i"(x=w541, y=w538) -> (x/y=w540:dbl[])
              n191 = Multiply "* J' * korr"(x=w548, y=w549) -> (x*y=w539:dbl[])
              n192 = Add(x=w539, y=w540) -> (x+y=w543:dbl[])
              n193 = Multiply(x=w565, y=w543) -> (x*y=w597:dbl[])
              n194 = Multiply(x=w598, y=w597) -> (x*y=w601:dbl[])
            }
          }
          "Untersetzung\nermittelt" <- w375
          n195 = local read "Übersetzung ermitteln aus"() -> (w358:T2)
          n196 = Quotient & Remainder(x=w361, y=500) -> (x-y*floor(x/y)=w363:i32)  [unwired: 1 out]
          n197 = Equal To 0? "aus Zündsignal?"(x=w358) -> (x = 0?=w374:bool)
          n198 = Equal To 0?(x=w363) -> (x = 0?=w362:bool)
          n199 = local read "Leistung"() -> (w333:bool)
          n200 = local read "Rollendrehzahl aufzeichnen"() -> (w335:bool)
          n201 = And(x=w375, y=w374) -> (x .and. y?=w373:bool)
          n202 = case shown="True" w362 {
            tunnel: w367 -> [_ w443]
            tunnel: w366 -> [_ w433]
            tunnel: w365 -> [_ w439]
            tunnel: w358 -> [_ w435]
            tunnel: "Rollenumfang [m]" -> [_ w442]
            tunnel: w356 -> [_ w432]
            frame False {
            }
            frame True {
              # "Skal-Y2"
              # "Skal-Y1"
              # "Skal-X"
              n203 = call "n2v (SubVI).vi"("Übersetzung ermitteln aus"=w435, "Array (Eingang)"=w443, "Rollenumfang [m]"=w442) -> ("Array (Ausgang)"=w436:dbl[])  [unwired: 7 in, 1 out]
              n204 = control-ref of="XY-Graph"() -> (w430:refnum<vi>)
              n205 = case shown="Standard" w435 {
                tunnel: [w448 w450] -> w434
                tunnel: w433 -> [w448 _]
                tunnel: w432 -> [_ w450]
                tunnel: [w448 w450] -> w431
                tunnel: [10.0 1000.0] -> w428
                frame Default {
                }
                frame "Vario (km/h)" {
                }
              }
              n206 = call "Scale_Graph_Y (SubVI).vi"("AktYSkl"=1, "Divisor"=w428, "Array"=w431, "Faktor"=1.8, "XYGraph (Eingang)"=w430) -> ()  [unwired: 7 in]
              n207 = call "Scale_Graph_Y (SubVI).vi"("AktYSkl"=0, "Divisor"=10.0, "Array"=w439, "Faktor"=1.0, "XYGraph (Eingang)"=w430) -> ()  [unwired: 7 in]
              n208 = Bundle("Array (Ausgang)"=w436, "Filtered X"=w434) -> (w444:T5)  [unwired: 1 in]
              n209 = Bundle("Array (Ausgang)"=w436, w439) -> (w445:cluster{"Array (Ausgang)":dbl[], dbl[]})  [unwired: 1 in]
              n210 = call "Scale_Graph_X (SubVI).vi"("Array"=w436, "Übersetzung ermitteln aus"=w435, "XYGraph (Eingang)"=w430) -> ()  [unwired: 9 in]
              n211 = Build Array(w445, w444) -> (w446:T6)
              n212 = local write "XY-Graph"(w446) -> ()
            }
          }
          n213 = Select(t=w372, s=w375, f=0.0) -> (s? t:f=→"Untersetzung":dbl)
          n214 = case shown="True" w373 {
            tunnel: w372 -> [_ w460]
            frame False {
            }
            frame True {
              n215 = local write "nKuWe/nRolle"(w460) -> ()
            }
          }
          n216 = Not(x=w335) -> (.not. x?=w334:bool)
          n217 = And(x=w333, y=w334) -> (x .and. y?=w332:bool)
          n218 = case shown="True" w332 {
            tunnel: [FALSE w459] -> w404
            tunnel: w403 -> [_ w458]
            frame False {
            }
            frame True {
              n219 = Greater Than 0?(x=w458) -> (x > 0?=w459:bool)
            }
          }
          n220 = local read "Start"() -> (w384:bool)
          n221 = Not(x=w384) -> (.not. x?=w327:bool)
          n222 = case shown="True" w327 {
            frame False {
            }
            frame True {
              n223 = property on="Lauf abgebrochen" class="Bool. (strikt)"("Value"=TRUE) -> ()  [unwired: 2 in, 2 out]
            }
          }
          n224 = Or(x=w404, y=w327) -> (x .or. y?=w407:bool)
        }
        n225 = VISA Clear(VISA resource name=w53, error in (no error)=w52) -> (VISA resource name out=w50:refnum<visa-resource-name>, error out=w54:errorcluster)
        n226 = VISA Close(VISA resource name=w50, error in (no error)=w54) -> ()  [unwired: 1 out]
        n227 = case shown="True" w68 {
          tunnel: w37 -> [_ w243]
          tunnel: w38 -> [_ w244]
          tunnel: w39 -> [_ w245]
          tunnel: w67 -> [_ w254]
          tunnel: w49 -> [_ w300]
          tunnel: w66 -> [_ w299]
          tunnel: w26 -> [_ w277]
          tunnel: w40 -> [_ w259]
          tunnel: w63 -> [_ w283]
          tunnel: w36 -> [_ w242]
          frame False {
          }
          frame True {
            w275 = 1
            w268 = 0
            w278 = 0.06
            n228 = Array Subset "P"(array=w245, length=w254) -> (w249:dbl[])  [unwired: 1 in]
            n229 = Array Subset "n"(array=w243, length=w254) -> (w247:dbl[])  [unwired: 1 in]
            n230 = Array Subset "M"(array=w244, length=w254) -> (w248:dbl[])  [unwired: 1 in]
            n231 = Array Subset "alpha"(array=w300, length=w254) -> (w301:dbl[])  [unwired: 1 in]
            n232 = Array Subset "nWelle"(array=w242, length=w254) -> (w246:dbl[])  [unwired: 1 in]
            n233 = property on="Ergebnis" class="Str"("Text.FontSize"=18) -> ()  [unwired: 2 in, 2 out]
            n234 = Array Size(array=w301) -> (size(s)=w302:i32)
            n235 = for {
              N: w302 -> [w321]
              tunnel: w300 -> [w318]
              tunnel: w243 -> [w315]
              tunnel: w299 -> [w312]
              tunnel: [w310] -> w291
              i -> [w316]
              stop <- w311 stop-if-true
              # "Beginn mit n(i)<nSchwelle &  a(i)<0 wegschneiden"
              n236 = Decrement(x=w321) -> (x-1=w320:i32)
              n237 = Subtract(x=w320, y=w316) -> (x-y=w310:i32)
              n238 = Index Array(array=w315, index=w310) -> (element=w314:dbl)
              n239 = Index Array(array=w318, index=w310) -> (element=w319:dbl)
              n240 = Less?(x=w314, y=w312) -> (x < y?=w313:bool)
              n241 = Less Or Equal To 0?(x=w319) -> (x <= 0?=w317:bool)
              n242 = And(x=w317, y=w313) -> (x .and. y?=w311:bool)
            }
            n243 = local read "Übersetzung ermitteln aus"() -> (w266:T2)
            n244 = Increment(x=w291) -> (x+1=w250:i32)
            n245 = Array Subset "nWelle"(array=w246, index=w250) -> (w251:dbl[])  [unwired: 1 in]
            n246 = Array Max & Min "nWelle_max [1/min]"(array=w251) -> (max value=w253:dbl)  [unwired: 3 out]
            n247 = Array Subset "n"(array=w247, index=w250) -> (w287:dbl[])  [unwired: 1 in]
            n248 = Array Subset "M"(array=w248, index=w250) -> (w265:dbl[])  [unwired: 1 in]
            n249 = Array Max & Min "Mmax"(array=w265) -> (max value=w264:dbl, max index (indices)=w288:i32)  [unwired: 2 out]
            n250 = Array Max & Min "nmax [1/min]"(array=w287) -> (max value=w262:dbl)  [unwired: 3 out]
            n251 = Array Subset "P"(array=w249, index=w250) -> (w255:dbl[])  [unwired: 1 in]
            n252 = Index Array "n(Mmax)"(array=w287, index=w288) -> (element=w286:dbl)
            n253 = Array Max & Min "Pmax"(array=w255) -> (max value=w241:dbl, max index (indices)=w252:i32)  [unwired: 2 out]
            "Pmax" <- w241
            n254 = call "n2v (SubVI).vi"("Übersetzung ermitteln aus"=w266, "Array (Eingang)"=w287, "Rollenumfang [m]"=w277) -> ("Array (Ausgang)"=w257:dbl[], "Boolesch"=w279:bool)  [unwired: 7 in]
            n255 = Index Array "nWelle (Pmax)"(array=w251, index=w252) -> (element=w239:dbl)
            n256 = Index Array "n(Pmax)"(array=w287, index=w252) -> (element=w238:dbl)
            n257 = case shown="Standard" w266 {
              tunnel: [w306 w309] -> w256
              tunnel: w265 -> [w306 _]
              tunnel: w251 -> [_ w309]
              tunnel: w264 -> [w305 _]
              tunnel: [w305 w308] -> w263
              tunnel: w253 -> [_ w308]
              tunnel: [w304 w307] -> w240
              tunnel: w239 -> [_ w307]
              tunnel: w238 -> [w304 _]
              frame Default {
              }
              frame "Vario (km/h)" {
              }
            }
            "n(Pmax)" <- w240
            n258 = Divide(x=w262, y=w283) -> (x/y=w298:dbl)
            n259 = local read "Lufttemperatur [°C]"() -> (w260:dbl)
            n260 = Format Into String(format string="%.1f PS" ("Format-String"), w241) -> (resulting string=→"Pmax":string)  [unwired: 2 in, 1 out]
            n261 = local read "Luftdruck [mbar]"() -> (w261:dbl)
            n262 = local read "Strecke [m]"() -> (w236:dbl)
            n263 = Compound Arithmetic op=MULTIPLY "v(Pmax)"(w238, w277, w278) -> (w284:dbl)
            n264 = Compound Arithmetic op=MULTIPLY "vmax"(w298, w277, w278) -> (w258:dbl)
            n265 = Format Date/Time String(time format string (%c)="%x %H:%M") -> (date/time string=w237:string)  [unwired: 2 in]
            "Datum+Zeit" <- w237
            n266 = Format Into String(format string="%.1f PS bei %d 1/min   |   %.1f Nm bei %d 1/min   |   vmax %d km/h\\nDIN 70020 k =%.3f (%d \\B0C, %d mbar)   |   %.0f m\\n%s" ("Format-String"), w241, w238, w264, w286, w258, w259, w260, w261, w236, w237) -> (resulting string=w282:string)  [unwired: 2 in, 1 out]
            n267 = Format Into String(format string="%.1f PS bei %d km/h, %d 1/min   |   vmax %d km/h\\nDIN 70020 k =%.3f (%d \\B0C, %d mbar)   |   %.0f m\\n%s" ("Format-String"), w241, w284, w239, w258, w259, w260, w261, w236, w237) -> (resulting string=w280:string)  [unwired: 2 in, 1 out]
            n268 = Bundle("Array (Ausgang)"=w257, w255) -> (w290:cluster{"Array (Ausgang)":dbl[], dbl[]})  [unwired: 1 in]
            n269 = Bundle("Array (Ausgang)"=w257, w256) -> (w289:cluster{"Array (Ausgang)":dbl[], dbl[]})  [unwired: 1 in]
            n270 = control-ref of="XY-Graph"() -> (w276:refnum<vi>)
            n271 = Select(t=w280, s=w279, f=w282) -> (s? t:f=→"Ergebnis":string)
            n272 = Multiply(x=1.8, y=w263) -> (x*y=w274:dbl)
            n273 = Build Array(w290, w289) -> (→"XY-Graph":cluster{"Array (Ausgang)":dbl[], dbl[]}[])
            n274 = property on="Pmax" class="Str"("Text.FontSize"=48) -> ()  [unwired: 2 in, 2 out]
            n275 = property on="Eigenschaftsknoten" class="XYGraph (strikt)"(reference=w276, "ActYScl"=w268, "YScale.ScaleFit"=w275, "XScale.ScaleFit"=w275, "ActYScl"=w275, "YScale.Maximum"=w274, "YScale.Minimum"=w268) -> (reference out=w272:refnum<vi>)  [unwired: 1 in, 1 out]
            n276 = property on="Eigenschaftsknoten" class="XYGraph (strikt)"(reference=w272, "ActYScl"=w268) -> (reference out=w269:refnum<vi>, "YScale.Maximum"=w271:dbl)  [unwired: 1 in, 1 out]
            n277 = Add(x=w271, y=3.0) -> (x+y=w267:dbl)
            n278 = property on="Eigenschaftsknoten" class="XYGraph (strikt)"(reference=w269, "ActYScl"=w268, "YScale.Maximum"=w267) -> ()  [unwired: 1 in, 2 out]
          }
        }
        n279 = flat-sequence {
          tunnel: w62 -> [w189]
          tunnel: w25 -> [w181]
          tunnel: w26 -> [w182]
          tunnel: w63 -> [w190]
          tunnel: w64 -> [w183]
          tunnel: w65 -> [w191]
          tunnel: [w191] -> w86
          tunnel: [w183] -> w85
          tunnel: [w190] -> w84
          tunnel: [w182] -> w83
          tunnel: [w181] -> w82
          tunnel: [w189] -> w81
          tunnel: [w185] -> w51
          tunnel: w50 -> [w185]
          tunnel: [w184] -> w43
          tunnel: w42 -> [w184]
          tunnel: w86 -> [w230]
          tunnel: w85 -> [w229]
          tunnel: w84 -> [w228]
          tunnel: w83 -> [w227]
          tunnel: w82 -> [w226]
          tunnel: w81 -> [w225]
          tunnel: w51 -> [w210]
          tunnel: w43 -> [w205]
          frame #0 {
            w187 = FALSE ("Start [F1]")
            w188 = 0  # Aktivieren
            n280 = local write "Start"(w187) -> ()
            n281 = property on="Drucken" class="Bool. (strikt)"("DisabledEnum"=w188) -> ()  [unwired: 2 in, 2 out]
            n282 = property on="Übersetzung ermitteln aus" class="Enum (strikt)"("DisabledEnum"=w188) -> ()  [unwired: 2 in, 2 out]
            n283 = property on="Speichern" class="Bool. (strikt)"("DisabledEnum"=w188) -> ()  [unwired: 2 in, 2 out]
            n284 = property on="Konfiguration:" class="Bool. (strikt)"("DisabledEnum"=w188) -> ()  [unwired: 2 in, 2 out]
            n285 = property on="Ende" class="Bool. (strikt)"("DisabledEnum"=w188) -> ()  [unwired: 2 in, 2 out]
            n286 = property on="Untersetzung\nermittelt" class="Bool. (strikt)"("BoolText.Text"="GO" ("Boolescher Text.Text"), "Blinking"=w187) -> ()  [unwired: 2 in, 2 out]
            n287 = local write "Untersetzung\nermittelt"(w187) -> ()
          }
          frame #1 {
            w206 = dbl[] []
            # "Es können evtl. aus Datenspeicher noch mehrere Werte entfernt und für anderes verwendet \nwerden, da einige in diesem VI nicht beschrieben und evlt. auch in ReCalc nicht verwendet werden\n(ggf. in ReCalc prüfen ob das auch tatsächlich so ist)"
            n288 = local read "Überschrift Leistungsdiagramm"() -> (w193:string)
            n289 = local read "Datum+Zeit"() -> (w197:string)
            n290 = local read "Lufttemperatur [°C]"() -> (w217:dbl)
            n291 = local read "Luftdruck [mbar]"() -> (w216:dbl)
            n292 = local read "Gleitender Mittelwert"() -> (w219:u8)
            n293 = local read "Differenzenquotient"() -> (w218:u8)
            n294 = local read "Übersetzung ermitteln aus"() -> (w215:T2)
            n295 = local read "Verlustmoment M1 [Nm] bei n1"() -> (w202:dbl)
            n296 = local read "Verlustmoment M0 [Nm] bei n = 0"() -> (w203:dbl)
            n297 = Path To String(path="Auto-Pfad") -> (string=w200:string)
            n298 = local read "Rollenträgheit [kgm²]"() -> (w223:dbl)
            n299 = local read "Rollendrehzahl n1 [1/min]"() -> (w204:u16)
            n300 = local read "Messung Klimadaten"() -> (w212:bool)
            n301 = local read "Reifenumfang [m]"() -> (w220:dbl)
            n302 = local read "n vom Gas [1/min]"() -> (w213:u16)
            n303 = local read "Zündung [Imp/U]"() -> (w222:dbl)
            n304 = local read "v vom Gas [km/h]"() -> (w208:u16)
            n305 = local read "nKuWe/nRolle"() -> (w209:dbl)
            n306 = local read "Getriebe [1:]"() -> (w221:dbl)
            n307 = Concatenate Strings(w197, "|", w200) -> (w199:string)
            n308 = local read "Dauer [s]"() -> (w214:u8)
            n309 = local read "Rollengeber [Inkr/U]"() -> (w224:u16)
            n310 = local read "Strecke [m]"() -> (w196:dbl)
            n311 = Concatenate Strings("Fahrzeugdaten", "§$", w193) -> (w195:string)
            n312 = Bundle(w195, w199, "Rollengeber [Inkr/U]"=w224, "Rollenumfang [m]"=w227, "Rollenträgheit [kgm²]"=w223, "Zündung [Imp/U]"=w222, "Getriebe [1:]"=w221, "Reifenumfang [m]"=w220, "mean value"=w228, "Gleitender Mittelwert"=w219, "Differenzenquotient"=w218, u8 0, w230, "Strecke [m]"=w196, "Lufttemperatur [°C]"=w217, "Rollendrehzahl n1 [1/min]"=w204, "Luftdruck [mbar]"=w216, w229, w205, w206, w206, "Übersetzung ermitteln aus"=w215, "Dauer [s]"=w214, "Verlustmoment M0 [Nm] bei n = 0"=w203, "Verlustmoment M1 [Nm] bei n1"=w202, "n vom Gas [1/min]"=w213, w226, w225, "Messung Klimadaten"=w212, "VISA-Referenz (Ausgang)"=w210, "nKuWe/nRolle"=w209, "v vom Gas [km/h]"=w208) -> (→"Datenspeicher":T7)  [unwired: 1 in]
          }
          frame #2 {
            n313 = local read "Auto-Speichern"() -> (w233:bool)
            n314 = local read "Lauf abgebrochen"() -> (w232:bool)
            n315 = Not(x=w232) -> (.not. x?=w231:bool)
            n316 = And(x=w233, y=w231) -> (x .and. y?=w234:bool)
            n317 = case shown="True" w234 {
              frame False {
              }
              frame True {
                n318 = property on="Speichern" class="Bool. (strikt)"("Val(Sgnl)"=TRUE) -> ()  [unwired: 2 in, 2 out]
              }
            }
          }
        }
      }
    }
    n319 = Boolean To (0,1)(Boolean=w10) -> (0, 1=w11:i16)
    n320 = property on="Registerkarte 2" class="RKElem (strikt)"("Value"=w11) -> ()  [unwired: 2 in, 2 out]
    n321 = local read "Ende"() -> (w12:bool)
  }
  n322 = while {
    stop <- w733 stop-if-true
    n323 = Wait (ms)(milliseconds to wait=10) -> ()  [unwired: 1 out]
    n324 = local read "Übersetzung ermitteln aus"() -> (w731:T2)
    n325 = local read "Leistung"() -> (w732:bool)
    n326 = case shown="Standard" w731 {
      tunnel: [FALSE TRUE] -> w730
      frame Default {
      }
      frame "Vario (km/h)" {
      }
    }
    n327 = case shown="False" w732 {
      tunnel: w730 -> [w741 _]
      frame False {
        n328 = control-ref of="Welle\n[1/min]"() -> (w745:refnum<vi>)
        n329 = control-ref of="Hinterrad\n[km/h]"() -> (w744:refnum<vi>)
        n330 = control-ref of="Ende"() -> (w743:refnum<vi>)
        n331 = control-ref of="Leistung"() -> (w742:refnum<vi>)
        n332 = call "Tachomodus (SubVI).vi"("cvt"=w741, "Leistung"=w742, "Stopp"=w743, "Hinterrad"=w744, "Welle"=w745) -> ()  [unwired: 7 in]
      }
      frame True {
      }
    }
    n333 = case shown="True" "Rollendrehzahl aufzeichnen" {
      frame False {
      }
      frame True {
        n334 = control-ref of="Rollendrehzahl aufzeichnen"() -> (w737:refnum<vi>)
        n335 = control-ref of="Ende"() -> (w736:refnum<vi>)
        n336 = control-ref of="Cyclecounter"() -> (w735:refnum<vi>)
        n337 = control-ref of="dT"() -> (w734:refnum<vi>)
        n338 = control-ref of="n(Rolle) [1/min]"() -> (w738:refnum<vi>)
        n339 = call "Rollendrehzahl (SubVI).vi"("dT(Rolle) (Eingang)"=w734, "Cyclecounter"=w735, "Stop"=w736, "Rollendrehzahl aufzeichnen"=w737, "n(Rolle) (Eingang)"=w738) -> ()  [unwired: 7 in]
      }
    }
    n340 = local read "Ende"() -> (w733:bool)
  }
  n341 = flat-sequence {
    frame #0 {
      n342 = local read "Datenspeicher"() -> (w764:T3)
      n343 = call <vilib>:"Application Directory.vi"() -> ("Application Directory"=w786:path)
      n344 = Build Path(base path=w786, name or relative path="Konfig.xml") -> (appended path=w766:path)
      n345 = call "LoadCluster(SubVI)2.0.5.vi"("Datenspeicher"=w764, "XML File Path"=w766) -> ("Value"=w765:T3)  [unwired: 7 in, 2 out]
      n346 = property on="Datenspeicher" class="Cluster (strikt)"("Value"=w765) -> ()  [unwired: 2 in, 2 out]
      n347 = Unbundle(w765) -> ("Fahrzeugdaten"=w749:string, "Auto-Pfad"=w757:string, "Rolle [Inkr/U]"=w784:u16, "Rollenumfang [m]"=w783:dbl, "Rollenträgheit [kgm²]"=w782:dbl, "Zündung [Imp/U]"=w781:dbl, "Getriebe [1:]"=w780:dbl, "Reifenumfang [m]"=w779:dbl, "element"=w770:dbl, "Gl. Mittelwert"=w778:u8, "Differenzenquotient"=w777:u8, "Lufttemperatur [°C]"=w776:dbl, "Mv: n1 [1/min]"=w760:dbl, "Luftdruck [mbar]"=w775:dbl, "Übersetzung ermitteln aus"=w772:u8, "[s]"=w774:dbl, "Mv: M0 [Nm]"=w762:dbl, "Mv: M1 [Nm]"=w763:dbl, "n vom Gas [1/min]"=w773:dbl, "Boolesch"=w771:bool, "Serielle Schnittstelle"=w769:refnum<visa-resource-name>, "nKuWe/nRolle"=w768:dbl, "v vom Gas [km/h]"=w767:dbl)  [unwired: 9 out]
      n348 = property on="Dauer [s]" class="DigWert (strikt)"("Value"=w774) -> ()  [unwired: 2 in, 2 out]
      n349 = property on="Rollengeber [Inkr/U]" class="DigWert (strikt)"("Value"=w784) -> ()  [unwired: 2 in, 2 out]
      n350 = property on="Rollenumfang [m]" class="DigWert (strikt)"("Value"=w783) -> ()  [unwired: 2 in, 2 out]
      n351 = property on="Rollenträgheit [kgm²]" class="DigWert (strikt)"("Value"=w782) -> ()  [unwired: 2 in, 2 out]
      n352 = property on="Zündung [Imp/U]" class="DigWert (strikt)"("Value"=w781) -> ()  [unwired: 2 in, 2 out]
      n353 = property on="Getriebe [1:]" class="DigWert (strikt)"("Value"=w780) -> ()  [unwired: 2 in, 2 out]
      n354 = property on="Reifenumfang [m]" class="DigWert (strikt)"("Value"=w779) -> ()  [unwired: 2 in, 2 out]
      n355 = property on="nKuWe/nRolle" class="DigWert (strikt)"("Value"=w770) -> ()  [unwired: 2 in, 2 out]
      n356 = property on="Gleitender Mittelwert" class="DigWert (strikt)"("Value"=w778) -> ()  [unwired: 2 in, 2 out]
      n357 = property on="Differenzenquotient" class="DigWert (strikt)"("Value"=w777) -> ()  [unwired: 2 in, 2 out]
      n358 = property on="Lufttemperatur [°C]" class="DigWert (strikt)"("Value"=w776) -> ()  [unwired: 2 in, 2 out]
      n359 = property on="Luftdruck [mbar]" class="DigWert (strikt)"("Value"=w775) -> ()  [unwired: 2 in, 2 out]
      n360 = property on="Übersetzung ermitteln aus" class="Enum (strikt)"("Val(Sgnl)"=w772) -> ()  [unwired: 2 in, 2 out]
      n361 = property on="n vom Gas [1/min]" class="DigWert (strikt)"("Value"=w773) -> ()  [unwired: 2 in, 2 out]
      n362 = property on="Messung Klimadaten" class="Bool. (strikt)"("Val(Sgnl)"=w771) -> ()  [unwired: 2 in, 2 out]
      n363 = local write "Serielle Schnittstelle"(w769) -> ()
      n364 = property on="nKuWe/nRolle" class="DigWert (strikt)"("Value"=w768) -> ()  [unwired: 2 in, 2 out]
      n365 = property on="v vom Gas [km/h]" class="DigWert (strikt)"("Value"=w767) -> ()  [unwired: 2 in, 2 out]
      n366 = property on="Verlustmoment M0 [Nm] bei n = 0" class="DigWert (strikt)"("Value"=w762) -> ()  [unwired: 2 in, 2 out]
      n367 = property on="Verlustmoment M1 [Nm] bei n1" class="DigWert (strikt)"("Value"=w763) -> ()  [unwired: 2 in, 2 out]
      n368 = Max & Min(x=1, y=w760) -> (max(x,y)=w759:dbl)  [unwired: 1 out]
      n369 = Search/Split String "führendes Datum+Zeit wegschneiden"(string=w757, search string/char (-)="|") -> (substring before match=w752:string, match + rest of string=w755:string)  [unwired: 1 in, 1 out]
      n370 = Search/Split String "führende Fahrzeugdaten wegschneiden"(string=w749, search string/char (-)="§$") -> (substring before match=w747:string, match + rest of string=w748:string)  [unwired: 1 in, 1 out]
      n371 = property on="Rollendrehzahl n1 [1/min]" class="DigWert (strikt)"("Value"=w759) -> ()  [unwired: 2 in, 2 out]
      n372 = String Subset(string=w755, offset (0)=1) -> (substring=w753:string)  [unwired: 1 in]
      n373 = String Subset(string=w748, offset (0)=2) -> (substring=w746:string)  [unwired: 1 in]
      n374 = String To Path(string=w753) -> (path=w758:path)
      n375 = property on="Fahrzeugdaten" class="Str"("Value"=w747) -> ()  [unwired: 2 in, 2 out]
      n376 = property on="Überschrift Leistungsdiagramm" class="Str"("Value"=w746) -> ()  [unwired: 2 in, 2 out]
      n377 = property on="Auto-Pfad" class="Pfad"("Value"=w758) -> ()  [unwired: 2 in, 2 out]
      n378 = property on="Datum+Zeit" class="Str"("Value"=w752) -> ()  [unwired: 2 in, 2 out]
    }
    frame #1 {
      w793 = 2  # Deaktivieren
      w795 = 0.0  # Graphen löschen
      n379 = local read "Serielle Schnittstelle"() -> (w791:refnum<visa-resource-name>)
      n380 = property on="Füllstand Lesepuffer" class="Schieber (strikt)"("Scale.Maximum"=100) -> ()  [unwired: 2 in, 2 out]
      n381 = property on="Frontpanel-Position" class="Bereich"("Origin"=T8 {"Horizontal"=8, "Vertical"=6}) -> ()  [unwired: 2 in, 2 out]
      n382 = property on="Drucken" class="Bool. (strikt)"("DisabledEnum"=w793) -> ()  [unwired: 2 in, 2 out]
      n383 = property on="Speichern" class="Bool. (strikt)"("DisabledEnum"=w793) -> ()  [unwired: 2 in, 2 out]
      n384 = Build Array(w795) -> (w794:dbl[])
      n385 = VISA Clear(VISA resource name=w791) -> (VISA resource name out=w790:refnum<visa-resource-name>, error out=w789:errorcluster)  [unwired: 1 in]
      n386 = property on="Untersetzung-Graph" class="SVDiagr (strikt)"("History Data"=w794) -> ()  [unwired: 2 in, 2 out]
      n387 = VISA Close(VISA resource name=w790, error in (no error)=w789) -> (error out=w788:errorcluster)
      n388 = case shown="Kein Fehler" w788 {
        tunnel: [T4."Enabled" ("Deaktiviert") T4."Disabled and Grayed Out" ("Deaktiviert")] -> w787
        frame No Error {
        }
        frame Error {
        }
      }
      n389 = property on="Start" class="Bool. (strikt)"("DisabledEnum"=w787) -> ()  [unwired: 2 in, 2 out]
    }
  }
  n390 = while {
    stop <- w802 stop-if-true
    n391 = event shown="[1] \"Drucken\": Wertänderung" {
      selector: _ -> [_ _ _ _ _ _ _ _ _ _ _ _]
      dyn-events: _ -> [_ _ _ _ _ _ _ _ _ _ _ _]
      timeout: _ -> [_ _ _ _ _ _ _ _ _ _ _ _]
      tunnel: [_ _ _ TRUE _ _ _ _ _ _ _ _] -> w802
      event "Konfiguration:": Value Change {
        n392 = event-data() -> ("OldVal"=w804:bool)  [unwired: 1 in, 5 out]
        n393 = flat-sequence {
          tunnel: [w842] -> w805
          tunnel: w804 -> [w842]
          tunnel: w805 -> [w843]
          frame #0 {
            n394 = property on="Datenspeicher" class="Cluster (strikt)"() -> ("Value"=w841:T3)  [unwired: 2 in, 2 out]
            n395 = call "LoadCluster(SubVI)2.0.5.vi"("Datenspeicher"=w841) -> ("Value"=w840:T3)  [unwired: 8 in, 2 out]
            n396 = Unbundle(w840) -> ("Fahrzeugdaten"=w807:string, "Auto-Pfad"=w815:string, "Rolle [Inkr/U]"=w839:u16, "Rollenumfang [m]"=w838:dbl, "Rollenträgheit [kgm²]"=w837:dbl, "Zündung [Imp/U]"=w836:dbl, "Getriebe [1:]"=w835:dbl, "Reifenumfang [m]"=w834:dbl, "Gl. Mittelwert"=w833:u8, "Differenzenquotient"=w832:u8, "Lufttemperatur [°C]"=w831:dbl, "Mv: n1 [1/min]"=w812:dbl, "Luftdruck [mbar]"=w830:dbl, "Übersetzung ermitteln aus"=w827:u8, "[s]"=w829:dbl, "Mv: M0 [Nm]"=w823:dbl, "Mv: M1 [Nm]"=w822:dbl, "n vom Gas [1/min]"=w828:dbl, "Boolesch"=w826:bool, "nKuWe/nRolle"=w825:dbl, "v vom Gas [km/h]"=w824:dbl)  [unwired: 11 out]
            n397 = property on="Dauer [s]" class="DigWert (strikt)"("Value"=w829) -> ()  [unwired: 2 in, 2 out]
            n398 = property on="Übersetzung ermitteln aus" class="Enum (strikt)"("Val(Sgnl)"=w827) -> ()  [unwired: 2 in, 2 out]
            n399 = property on="Rollengeber [Inkr/U]" class="DigWert (strikt)"("Value"=w839) -> ()  [unwired: 2 in, 2 out]
            n400 = property on="Rollenumfang [m]" class="DigWert (strikt)"("Value"=w838) -> ()  [unwired: 2 in, 2 out]
            n401 = property on="Rollenträgheit [kgm²]" class="DigWert (strikt)"("Value"=w837) -> ()  [unwired: 2 in, 2 out]
            n402 = property on="Zündung [Imp/U]" class="DigWert (strikt)"("Value"=w836) -> ()  [unwired: 2 in, 2 out]
            n403 = property on="Getriebe [1:]" class="DigWert (strikt)"("Value"=w835) -> ()  [unwired: 2 in, 2 out]
            n404 = property on="Reifenumfang [m]" class="DigWert (strikt)"("Value"=w834) -> ()  [unwired: 2 in, 2 out]
            n405 = property on="Gleitender Mittelwert" class="DigWert (strikt)"("Value"=w833) -> ()  [unwired: 2 in, 2 out]
            n406 = property on="Differenzenquotient" class="DigWert (strikt)"("Value"=w832) -> ()  [unwired: 2 in, 2 out]
            n407 = property on="Lufttemperatur [°C]" class="DigWert (strikt)"("Value"=w831) -> ()  [unwired: 2 in, 2 out]
            n408 = property on="Luftdruck [mbar]" class="DigWert (strikt)"("Value"=w830) -> ()  [unwired: 2 in, 2 out]
            n409 = property on="n vom Gas [1/min]" class="DigWert (strikt)"("Value"=w828) -> ()  [unwired: 2 in, 2 out]
            n410 = property on="Messung Klimadaten" class="Bool. (strikt)"("Val(Sgnl)"=w826) -> ()  [unwired: 2 in, 2 out]
            n411 = property on="nKuWe/nRolle" class="DigWert (strikt)"("Value"=w825) -> ()  [unwired: 2 in, 2 out]
            n412 = property on="v vom Gas [km/h]" class="DigWert (strikt)"("Value"=w824) -> ()  [unwired: 2 in, 2 out]
            n413 = property on="Verlustmoment M1 [Nm] bei n1" class="DigWert (strikt)"("Value"=w822) -> ()  [unwired: 2 in, 2 out]
            n414 = property on="Verlustmoment M0 [Nm] bei n = 0" class="DigWert (strikt)"("Value"=w823) -> ()  [unwired: 2 in, 2 out]
            n415 = Search/Split String "führende Fahrzeugdaten wegschneiden"(string=w807, search string/char (-)="§$") -> (substring before match=w806:string, match + rest of string=w809:string)  [unwired: 1 in, 1 out]
            n416 = Search/Split String "führendes Datum+Zeit wegschneiden"(string=w815, search string/char (-)="|") -> (substring before match=w816:string, match + rest of string=w819:string)  [unwired: 1 in, 1 out]
            n417 = Max & Min(x=1, y=w812) -> (max(x,y)=w814:dbl)  [unwired: 1 out]
            n418 = String Subset(string=w809, offset (0)=2) -> (substring=w808:string)  [unwired: 1 in]
            n419 = String Subset(string=w819, offset (0)=1) -> (substring=w817:string)  [unwired: 1 in]
            n420 = String To Path(string=w817) -> (path=w821:path)
            n421 = property on="Rollendrehzahl n1 [1/min]" class="DigWert (strikt)"("Value"=w814) -> ()  [unwired: 2 in, 2 out]
            n422 = property on="Überschrift Leistungsdiagramm" class="Str"("Value"=w808) -> ()  [unwired: 2 in, 2 out]
            n423 = property on="Datum+Zeit" class="Str"("Value"=w816) -> ()  [unwired: 2 in, 2 out]
            n424 = property on="Fahrzeugdaten" class="Str"("Value"=w806) -> ()  [unwired: 2 in, 2 out]
            n425 = property on="Auto-Pfad" class="Pfad"("Value"=w821) -> ()  [unwired: 2 in, 2 out]
          }
          frame #1 {
            n426 = property on="Konfiguration:" class="Bool. (strikt)"("Value"=w843) -> ()  [unwired: 2 in, 2 out]
          }
        }
      }
      event "Drucken": Value Change {
        n427 = event-data() -> ("OldVal"=w844:bool)  [unwired: 1 in, 5 out]
        n428 = flat-sequence {
          tunnel: [w850] -> w845
          tunnel: w844 -> [w850]
          tunnel: w845 -> [w851]
          frame #0 {
            n429 = control-ref of="Fahrzeugdaten"() -> (w848:refnum<vi>)
            n430 = control-ref of="Ergebnis"() -> (w847:refnum<vi>)
            n431 = control-ref of="Überschrift Leistungsdiagramm"() -> (w846:refnum<vi>)
            n432 = control-ref of="XY-Graph"() -> (w849:refnum<vi>)
            n433 = call "printgraph_V0.01.vi"("Überschrift"=w846, "Ergebnis"=w847, "Fahrzeugdaten"=w848, "XYGraph (Eingang)"=w849) -> ()  [unwired: 8 in]
          }
          frame #1 {
            n434 = property on="Drucken" class="Bool. (strikt)"("Value"=w851) -> ()  [unwired: 2 in, 2 out]
          }
        }
      }
      event "Speichern": Value Change {
        n435 = event-data() -> ("OldVal"=w852:bool)  [unwired: 1 in, 5 out]
        n436 = flat-sequence {
          frame #0 {
            n437 = property on="Auto-Gespeichert" class="Bool. (strikt)"("Value"=FALSE) -> ()  [unwired: 2 in, 2 out]
            n438 = property on="Auto-Datei" class="Str"("Value"="") -> ()  [unwired: 2 in, 2 out]
          }
          frame #1 {
            n439 = local read "Auto-Pfad"() -> (w864:path)
            n440 = property on="Auto-Speichern" class="Bool. (strikt)"() -> ("Value"=w858:bool)  [unwired: 2 in, 2 out]
            n441 = call <vilib>:"Check if File or Folder Exists.vi"("path"=w864) -> ("file or folder exists?"=w863:bool, "dup path"=w860:path)  [unwired: 8 in, 1 out]
            n442 = Not(x=w863) -> (.not. x?=w862:bool)
            n443 = And(x=w858, y=w862) -> (x .and. y?=w861:bool)
            n444 = And(x=w858, y=w863) -> (x .and. y?=w855:bool)
            n445 = call "Meldung an Benutzer2"("Enable"=w861) -> ()  [unwired: 9 in, 2 out]
            n446 = case shown="True" w855 {
              tunnel: [path "" w880] -> w865
              tunnel: w860 -> [_ w879]
              tunnel: ["" w873] -> w856
              frame False {
              }
              frame True {
                n447 = Get Date/Time In Seconds() -> (seconds since 1Jan1904=w883:timestamp)
                n448 = local read "Pmax"() -> (w876:dbl)
                n449 = local read "n(Pmax)"() -> (w875:dbl)
                n450 = Path To String(path=w879) -> (string=w882:string)
                n451 = Format Into String(format string="%,; %.1f_%d.xml" ("Format-String"), w876, w875) -> (resulting string=w871:string)  [unwired: 2 in, 1 out]
                n452 = Format Date/Time String(time format string (%c)="%y%m%d_%H%M%S_", seconds (now)=w883) -> (date/time string=w872:string)  [unwired: 1 in]
                n453 = Concatenate Strings(w882, "\\", w872, w871) -> (w881:string)
                n454 = Concatenate Strings(w872, w871) -> (w873:string)
                n455 = String To Path(string=w881) -> (path=w880:path)
              }
            }
            n456 = control-ref of="Datenspeicher"() -> (w866:refnum<vi>)
            n457 = call "savecluster_V0.01.vi"("selected path"=w865, "Datenspeicher 2"=w866) -> ("Kein Fehler"=w859:bool)
            n458 = And(x=w855, y=w859) -> (x .and. y?=w857:bool)
            n459 = case shown="True" w857 {
              tunnel: w856 -> [_ w868]
              frame False {
              }
              frame True {
                n460 = property on="Auto-Gespeichert" class="Bool. (strikt)"("Value"=TRUE) -> ()  [unwired: 2 in, 2 out]
                n461 = property on="Auto-Datei" class="Str"("Value"=w868) -> ()  [unwired: 2 in, 2 out]
              }
            }
          }
        }
        n462 = local write "Speichern"(w852) -> ()
      }
      event "Ende": Value Change {
        w892 = 0.0 ("element")
        n463 = event-data() -> ("OldVal"=w890:bool)  [unwired: 1 in, 5 out]
        n464 = local read "Datenspeicher"() -> (w893:T3)
        n465 = flat-sequence {
          tunnel: w890 -> [w922]
          tunnel: [w922] -> w889
          frame #0 {
            n466 = Wait (ms)(milliseconds to wait=u32 200) -> ()  [unwired: 1 out]
          }
        }
        n467 = Unbundle By Name(w893) -> ("Auto-Pfad"=w884:string, "Rolle [Inkr/U]"=w914:u16, "Rollenumfang [m]"=w913:dbl, "Rollenträgheit [kgm²]"=w912:dbl, "Zündung [Imp/U]"=w911:dbl, "Getriebe [1:]"=w910:dbl, "Reifenumfang [m]"=w909:dbl, "Gl. Mittelwert"=w908:u8, "Differenzenquotient"=w907:u8, "Fahrzeugdaten"=w906:string, "Lufttemperatur [°C]"=w905:dbl, "Mv: n1 [1/min]"=w904:dbl, "Luftdruck [mbar]"=w902:dbl, "nRolle"=w903:dbl[], "Übersetzung ermitteln aus"=w901:u8, "[s]"=w900:dbl, "Mv: M0 [Nm]"=w899:dbl, "Mv: M1 [Nm]"=w898:dbl, "n vom Gas [1/min]"=w897:dbl, "Boolesch"=w896:bool, "Serielle Schnittstelle"=w891:refnum<visa-resource-name>, "nWelle"=w888:dbl[], "ArrayReserve1"=w886:dbl[], "ArrayReserve2"=w885:dbl[], "v vom Gas [km/h]"=w887:dbl)  [unwired: 3 out]
        n468 = call <vilib>:"Application Directory.vi"() -> ("Application Directory"=w917:path)
        n469 = local write "Ende"(w889) -> ()
        n470 = Bundle By Name(cluster=w893, "Auto-Pfad"=w884, "Rolle [Inkr/U]"=w914, "Rollenumfang [m]"=w913, "Rollenträgheit [kgm²]"=w912, "Zündung [Imp/U]"=w911, "Getriebe [1:]"=w910, "Reifenumfang [m]"=w909, "element"=0.0, "Gl. Mittelwert"=w908, "Differenzenquotient"=w907, "Fahrzeugdaten"=w906, "element"=w892, "element"=w892, "Lufttemperatur [°C]"=w905, "Mv: n1 [1/min]"=w904, "Luftdruck [mbar]"=w902, "nRolle"=w903, "Übersetzung ermitteln aus"=w901, "[s]"=w900, "Mv: M0 [Nm]"=w899, "Mv: M1 [Nm]"=w898, "n vom Gas [1/min]"=w897, "Boolesch"=w896, "Serielle Schnittstelle"=w891, "nWelle"=w888, "ArrayReserve1"=w886, "ArrayReserve2"=w885, "v vom Gas [km/h]"=w887) -> (w894:T3)
        n471 = Build Path(base path=w917, name or relative path="Konfig.xml") -> (appended path=w915:path)
        n472 = Flatten To XML(anything=w894) -> (xml string=w919:string)
        n473 = call-poly <vilib>:"Write to XML File.vi"("XML Input"=w919, "XML File Path"=w915) -> ("error out"=w918:errorcluster)  [unwired: 7 in, 2 out]
        n474 = case shown="Kein Fehler" w918 {
          frame No Error {
          }
          frame Error {
          }
        }
      }
      event "Serielle Schnittstelle": Value Change {
        n475 = event-data() -> ()  [unwired: 1 in, 6 out]
        n476 = property on="Start" class="Bool. (strikt)"("DisabledEnum"=T4."Enabled" ("Deaktiviert")) -> ()  [unwired: 2 in, 2 out]
      }
      event "Messung Klimadaten": Value Change {
        n477 = event-data() -> ("NewVal"=w924:bool)  [unwired: 1 in, 5 out]
        n478 = case shown="True" w924 {
          frame True {
            w925 = T4."Disabled and Grayed Out" ("Deaktiviert")
            n479 = property on="Lufttemperatur [°C]" class="DigWert (strikt)"("DisabledEnum"=w925) -> ()  [unwired: 2 in, 2 out]
            n480 = property on="Luftdruck [mbar]" class="DigWert (strikt)"("DisabledEnum"=w925) -> ()  [unwired: 2 in, 2 out]
          }
          frame False {
            w926 = T4."Enabled" ("Deaktiviert")
            n481 = property on="Lufttemperatur [°C]" class="DigWert (strikt)"("DisabledEnum"=w926) -> ()  [unwired: 2 in, 2 out]
            n482 = property on="Luftdruck [mbar]" class="DigWert (strikt)"("DisabledEnum"=w926) -> ()  [unwired: 2 in, 2 out]
          }
        }
      }
      event "Spenden": Value Change {
        n483 = event-data() -> ()  [unwired: 1 in, 6 out]
        n484 = case shown="True" "Spenden" {
          frame False {
          }
          frame True {
            w928 = "https://www.paypal.com/cgi-bin/webscr?cmd=_s-xclick&hosted_button_id=5HCL4L3EEXS64&source=url"  # GruA
            (unwired) "https://www.paypal.com/cgi-bin/webscr?cmd=_s-xclick&hosted_button_id=8SA7Y5J5P5N3W&source=url" ("URL")
            n485 = call-poly <vilib>:"Open URL in Default Browser.vi"("URL"=w928) -> ()  [unwired: 5 in, 2 out]
          }
        }
      }
      event "Recalc": Value Change {
        n486 = event-data() -> ("OldVal"=w931:bool)  [unwired: 1 in, 5 out]
        n487 = property on="Recalc" class="Bool. (strikt)"("Value"=w931) -> ()  [unwired: 2 in, 2 out]
        n488 = property on="Datenspeicher" class="Cluster (strikt)"() -> ("Value"=w929:T3)  [unwired: 2 in, 2 out]
        n489 = call "ReCalc_V2.00.vi"("Berechnen"=TRUE, "Datenspeicher"=w929) -> ()  [unwired: 3 in]
      }
      event "Übersetzung ermitteln aus": Value Change {
        n490 = event-data() -> ("NewVal"=w945:T2)  [unwired: 1 in, 5 out]
        n491 = case shown="\"Vario (km/h)\"" w945 {
          tunnel: [w961 w962 w964 w967] -> w946
          tunnel: [w961 w963 w964 w966] -> w941
          tunnel: [w961 w962 w965 w966] -> w932
          tunnel: [w961 w963 w965 w967] -> w940
          tunnel: [T4."Enabled" ("Deaktiviert") w962 w964 w966] -> w939
          frame "Vario (km/h)" {
            w961 = T4."Disabled and Grayed Out" ("Deaktiviert")
          }
          frame "nKuWe / nRolle" {
            w963 = T4."Enabled" ("Deaktiviert")
            w962 = T4."Disabled and Grayed Out" ("Deaktiviert")
          }
          frame "Zündsignal", Default {
            w965 = T4."Enabled" ("Deaktiviert")
            w964 = T4."Disabled and Grayed Out" ("Deaktiviert")
          }
          frame "Getriebe & Reifen" {
            w966 = T4."Disabled and Grayed Out" ("Deaktiviert")
            w967 = T4."Enabled" ("Deaktiviert")
          }
        }
        n492 = case shown="Standard" w945 {
          tunnel: ["n [1/min]" "M [Nm]"] -> w944
          tunnel: [200.0 14000.0] -> w943
          tunnel: ["v [km/h]" "n [1/min]"] -> w938
          tunnel: [14000.0 50.0] -> w937
          tunnel: [u32 16777216 w955] -> w935
          tunnel: [u32 16711680 w955] -> w934
          tunnel: [FALSE TRUE] -> w933
          frame "Vario (km/h)" {
          }
          frame Default {
            w955 = u32 9868950
          }
        }
        n493 = property on="Text Zündung" class="Str"("Text.TextColor"=w934) -> ()  [unwired: 2 in, 2 out]
        n494 = property on="Welle [1/min]" class="Drehknopf (strikt)"("Active Slider"=1, "FG Color"=w935) -> ()  [unwired: 2 in, 2 out]
        n495 = property on="Text Rolle" class="Str"("Visible"=w933) -> ()  [unwired: 2 in, 2 out]
        n496 = property on="XY-Graph" class="XYGraph (strikt)"("ActYScl"=1, "YScale.NameLbl.Text"=w944, "YScale.Maximum"=w937, "XScale.NameLbl.Text"=w938, "XScale.Maximum"=w943) -> ()  [unwired: 2 in, 2 out]
        n497 = property on="nKuWe/nRolle" class="DigWert (strikt)"("DisabledEnum"=w941) -> ()  [unwired: 2 in, 2 out]
        n498 = property on="v vom Gas [km/h]" class="DigWert (strikt)"("DisabledEnum"=w939) -> ()  [unwired: 2 in, 2 out]
        n499 = property on="n vom Gas [1/min]" class="DigWert (strikt)"("DisabledEnum"=w940) -> ()  [unwired: 2 in, 2 out]
        n500 = property on="Getriebe [1:]" class="DigWert (strikt)"("DisabledEnum"=w946) -> ()  [unwired: 2 in, 2 out]
        n501 = property on="Reifenumfang [m]" class="DigWert (strikt)"("DisabledEnum"=w946) -> ()  [unwired: 2 in, 2 out]
        n502 = property on="Zündung [Imp/U]" class="DigWert (strikt)"("DisabledEnum"=w932) -> ()  [unwired: 2 in, 2 out]
        n503 = property on="Dauer [s]" class="DigWert (strikt)"("DisabledEnum"=w932) -> ()  [unwired: 2 in, 2 out]
        n504 = property on="Filter Zündsignal" class="Bool. (strikt)"("DisabledEnum"=w932) -> ()  [unwired: 2 in, 2 out]
      }
      event "Reset Skalierung": Value Change {
        w972 = 0.0
        n505 = event-data() -> ()  [unwired: 1 in, 6 out]
        n506 = local read "Übersetzung ermitteln aus"() -> (w970:T2)
        n507 = case shown="\"Vario (km/h)\"" w970 {
          tunnel: [14000.0 200.0] -> w969
          tunnel: [50.0 14000.0] -> w968
          frame Default {
          }
          frame "Vario (km/h)" {
          }
        }
        n508 = property on="XY-Graph" class="XYGraph (strikt)"("XScale.Maximum"=w969, "XScale.Minimum"=w972, "ActYScl"=w972, "YScale.Maximum"=30.0, "YScale.Minimum"=w972, "ActYScl"=1, "YScale.Maximum"=w968, "YScale.Minimum"=w972) -> ()  [unwired: 2 in, 2 out]
      }
      event "Auto-Speichern": Value Change {
        n509 = event-data() -> ("NewVal"=w978:bool)  [unwired: 1 in, 5 out]
        n510 = case shown="True" w978 {
          frame False {
          }
          frame True {
            n511 = local read "Auto-Pfad"() -> (w981:path)
            n512 = call <vilib>:"Check if File or Folder Exists.vi"("path"=w981) -> ("file or folder exists?"=w979:bool)  [unwired: 8 in, 2 out]
            n513 = Not(x=w979) -> (.not. x?=w980:bool)
            n514 = call "Meldung an Benutzer"("Enable"=w980) -> ()  [unwired: 9 in, 2 out]
            n515 = local write "Auto-Speichern"(w979) -> ()
          }
        }
      }
      event "Fahrzeugdaten": Value Change {
        # "Fahrzeugdaten auf 3 Zeilen begrenzen\n(Recalc ist nur auf max. 3 Zeilen ausgelegt)"
        n516 = event-data() -> ("OldVal"=w984:string, "NewVal"=w985:string)  [unwired: 1 in, 4 out]
        n517 = Spreadsheet String To Array(delimiter (Tab)="\n", format string="%s", spreadsheet string=w985, array type (2D Dbl)=string[] []) -> (array=w987:string[])
        n518 = Array Size "Zeilenanzahl"(array=w987) -> (size(s)=w986:i32)
        n519 = Greater?(x=w986, y=3) -> (0:w983:bool)
        n520 = case shown="True" w983 {
          tunnel: w984 -> [_ w991]
          frame False {
          }
          frame True {
            n521 = flat-sequence {
              tunnel: w991 -> [w993]
              frame #0 {
                n522 = call "Meldung an Benutzer3"("Enable"=TRUE) -> ()  [unwired: 9 in, 2 out]
              }
              frame #1 {
                n523 = property on="Fahrzeugdaten" class="Str"("Value"=w993) -> ()  [unwired: 2 in, 2 out]
              }
            }
          }
        }
      }
    }
    n524 = property class="Anw"() -> ("App.Kind"=w800:T9)  [unwired: 2 in, 2 out]
    n525 = Greater?(x=w800, y=1) -> (0:w801:bool)
    n526 = case shown="True" w801 {
      tunnel: w802 -> [_ w803]
      frame False {
      }
      frame True {
        n527 = Quit LabVIEW(quit? (T)=w803) -> ()
      }
    }
  }
  n528 = property on="Auto-Speichern" class="Bool. (strikt)"("Value"=w2) -> ()  [unwired: 2 in, 2 out]
  "Text Zündung" <- "Zündung"
  "Text Rolle" <- "Rolle"
  "Auto-Gespeichert" <- w2
  "Auto-Datei" <- ""
